vi "Abgleich_Finetuning.vi"(0 "DAQ Settings":T1={"sampling rate [Hz]"=50000.0, "actual update rate"=50000.00001018634, "output physical channel"="SOUNDACQ/ao0", "input channel (stimulus)"="SOUNDACQ/ai0", "propagation delay [samples]"=133, "input channel (response)"="SOUNDACQ/ai1"} {"propagation delay [samples]" min=1 step=1; "actual update rate" format="%.2f"; "sampling rate [Hz]" format="%.2f"}, 1 "Soll_Pegel(dBSPL)":i32=-1, 5 "FRF Settings":T3={"window"=1, "block size"=1000, "view"={"dB On"=TRUE, "unwrap phase"=FALSE, "convert to degree"=TRUE}, "averaging parameters"={"averaging mode"=enum."RMS averaging", "weighting mode"=enum."Exponential", "number of averages"=2, "linear mode"=enum."One shot"}, "restart averaging"=FALSE} {"averaging parameters"."number of averages" min=1 step=1; "block size" min=128; "window" items=["None"=0, "Hanning"=1, "Hamming"=2, "Blackman-Harris"=3, "Exact Blackman"=4, "Blackman"=5, "Flat Top"=6, "4 Term B-Harris "=7, "7 Term B-Harris"=8, "Low Sidelobe"=9, "Force - Exponential"=10, "Blackman Nuttall"=11, "Triangle"=30, "Bartlett-Hanning"=31, "Bohman"=32, "Parzen"=33, "Welch"=34, "Kaiser"=60, "Dolph-Chebyshev"=61, "Gaussian"=62]}, 7 "frequency":dbl=1000.0, 9 "sensitivity(mV/Pa)":dbl=336.0, 11 "error in":errorcluster, 12 "Start_Amplitude(V)":dbl=0.605 min=0.0 format="%.3f") -> (4 "End_Amplitude(V)":dbl=0.605 min=0.0 format="%.3f", 6 "Ist_Pegel(dBSPL)":dbl=94.02694316227692, 8 "detected fund. amp.":dbl=0.47778380964100664 format="%.5f", 15 "error out":errorcluster)   [LabVIEW 2018]
uses:
  <vilib>/addons/_NISVFA/_Shared subVIs/Controls/svc_Window [Dual FFT].ctl
  <vilib>/DAQmx/write.llb/DAQmx Write (Analog 1D DBL 1Chan NSamp).vi
  <vilib>/DAQmx/read.llb/DAQmx Read (Analog 1D Wfm NChan NSamp).vi
  <vilib>/DAQmx/create/channels.llb/DAQmx Create Channel (AI-Voltage-Basic).vi
  <vilib>/DAQmx/configure/timing.llb/DAQmx Timing (Sample Clock).vi
  <vilib>/DAQmx/create/channels.llb/DAQmx Create Channel (AO-Voltage-Basic).vi
  <vilib>/DAQmx/configure/trigger.llb/DAQmx Start Trigger (Digital Edge).vi
  <vilib>/DAQmx/miscellaneous.llb/DAQmx Fill In Error Info.vi
  <vilib>/addons/_NISVFA/_Baseband FFT/SVFA Frequency Response (1x1) (Mag-Phase).vi
  <vilib>/addons/Sound and Vibration/svt_Distortion/SVT THD and Harmonic Components (Time) (1 Ch).vi
  <vilib>/addons/_NISVFA/_Baseband FFT/SVFA Power Spectrum (1 Ch).vi
  <vilib>/Analysis/NI_AALBase.lvlib
  <vilib>/addons/Sound and Vibration/svt_Distortion/SoundVib_Distortion.lvlib
  <resource>/objmgr/daqmx.rc
panel:
  out "fr1000Hz":dbl(graph)=999.9999374706828
  out "mean":dbl=0.501952560805785
  out "standard deviation":dbl=0.010795190304670955
  out "Array":u32[](array[numeric])
  out "Ist_Pegel(dBSPL) Time Chart":cluster{dbl[], dbl[]}[](graph)
  in  "Coh Faktor Thresold":dbl=999.98 format="%#_10g"
  out "Filtered FR_Time Chart":cluster{dbl[], dbl[]}(graph)
  out "Big Sound Disturbances detected":i32=1
  out "Sound Pressure (Pa)":dbl=1.0054886063639832
  in  "swept sine settings":enum32{"DAQ Settings", "FRF Settings"}(tab)
  in  "input channel (response)":tag="SOUNDACQ/ai1"
  in  "propagation delay [samples]":i32=133 min=1 step=1
  in  "input channel (stimulus)":tag="SOUNDACQ/ai0"
  in  "output physical channel":tag="SOUNDACQ/ao0"
  out "actual update rate":dbl=50000.00001018634 format="%.2f"
  in  "sampling rate [Hz]":dbl=50000.0 format="%.2f"
  out "averages completed":dbl=4358.0
  in  "restart averaging":bool
  in  "averaging parameters":T4={"averaging mode"=enum."RMS averaging", "weighting mode"=enum."Exponential", "number of averages"=2, "linear mode"=enum."One shot"} {"number of averages" min=1 step=1}
  in  "view":T5={"dB On"=TRUE, "unwrap phase"=FALSE, "convert to degree"=TRUE}
  in  "block size":i32=1000 min=128
  in  "window":T2=1 items=["None"=0, "Hanning"=1, "Hamming"=2, "Blackman-Harris"=3, "Exact Blackman"=4, "Blackman"=5, "Flat Top"=6, "4 Term B-Harris "=7, "7 Term B-Harris"=8, "Low Sidelobe"=9, "Force - Exponential"=10, "Blackman Nuttall"=11, "Triangle"=30, "Bartlett-Hanning"=31, "Bohman"=32, "Parzen"=33, "Welch"=34, "Kaiser"=60, "Dolph-Chebyshev"=61, "Gaussian"=62]
  in  "Tab Control":enum32{"Getting Started", "Time Record", "FRF"}(tab)=enum."FRF"
  in  "Getting Started Text":string="GETTING STARTED\n\nThis VI measures the Frequency Response Function (FRF) of a device under test (DUT).  It generates a broadband stimulus signal to excite the DUT.  The magnitude and phase of the DUT output are compared to the stimulus signal to calculate the FRF.  \n\nRefer to the wiring diagram to physically connect the DSA or DAQ device to the DUT.  This example uses two analog input channels and one analog output channel.  Note that the analog output is connected to both the DUT input and to the first analog input channel on the measurement device.  \n\nThe wiring diagram assumes that you use the default channel settings.  If you change the channel settings in the VI front panel you should adjust the physical connections appropriately.\n\nNI strongly recommends that you take precautions to limit the effects of out-of-band aliasing in your frequency domain measurements.  DSA devices use transparent digital and analog hardware filtering to eliminate aliased input and output frequencies.  Multifunction DAQ devices are more susceptible to the effects of aliased frequencies.  If you are using a non-DSA measurement device, we recommend addressing potential aliasing through high sampling rates, built-in analog filters on S Series devices, and/or external analog filters.\n\n\nKEY PARAMETERS\n\nDAQ Configuration:  device propagation delay [samples]\n\nThis parameter quantifies the time, measured in sample intervals, between when a sample of data is generated on analog output and when it is read on the analog input.  Common sources of delay are analog or digital filters and propagation time for acoustical or mechanical signals.  The combined delay of the digital anti-aliasing and anti-imaging filters on the NI PCI-4451 and PCI-4551 devices is approximately 77 samples.  When using a multifunction E Series or S Series device, we recommend entering a delay of 1 sample.  An easy way to determine this delay for any given measurement system is to run SVT Measure Propagation Delay.vi.  This VI is available from the LabVIEW Functions palette under Sound and Vibration >> Calibration.\n\n\nSource Settings:  signal type\n\nThis control allows you to specify the type of stimulus signal you would like to generate.  All of the available signal sources are broadband stimuli with frequency content ranging from just above DC to the value specified in the \"Maximum Frequency of Interest\" control.  Note that if you use the \"Chirp\" or \"Frequency flat chirp\" signal types, you should select \"None\" for the window type.\n\nSource Settings:  maximum frequency of interest [Hz]\n\nThis setting controls the sampling rate for input and output.  The sampling rate is 2.5 times the value of this control.  Reducing the maximum frequency of interest may help if you encounter issues of data transfer bandwidth.\n\nMeasurement Settings:  frequency resolution [Hz]\n\nThis setting controls the width of a single frequency bin in the frequency response measurement.  Improving the frequency resolution requires more data points per average. Thus, the acquisition block size increases with finer frequency resolutions.  Improving (i.e. reducing) the frequency resolution may help if you encounter issues of data transfer bandwidth. \n\nMeasurement Settings:  window\n\nThis setting controls the time-domain window applied to the input signals before the frequency response function is calculated.  If you use the \"Chirp\" or \"Frequency flat chirp\" excitation types, you should not apply a window.\n\n\nMeasurement Settings:  settle time [s]\n\nThis control allows you to specify a time interval between when the stimulus generation starts and when the measurement actually begins. This time interval will be coerced to an integer number of data blocks.  If your DUT has a significant transient response to the start of a stimulus signal, select the appropriate settle time to allow this transient response to pass.\n"
  out "time record 2":waveform(dbl)[](graph)=[{"t0"=timestamp(3564665204.4424295 s since 1904-01-01), "dt"=1.9999999995925458e-05, "Y"=array[1000 elements], "attributes"=variant("NI_ChannelName"=variant(string "stimulus"), "NI_UnitDescription"=variant(string "Volts"))}, {"t0"=timestamp(3564665204.4424295 s since 1904-01-01), "dt"=1.9999999995925458e-05, "Y"=array[1000 elements], "attributes"=variant("NI_ChannelName"=variant(string "response"), "NI_UnitDescription"=variant(string "Volts"))}]
  out "Waveform Graph":dbl[](graph)=[0.0, 0.07582660630640407, 0.15045738173473716, 0.22271535437423018, 0.29146097283153777, 0.35561007763694624, 0.4141509990868567, 0.4661605118793525, 0.5108183949287192, 0.5474203667419418, 0.5753891923585679, 0.5942837866908567, 0.6038061706991042, 0.6038061706991044, 0.5942837866908566, 0.5753891923585679, 0.5474203667419417, 0.510818394928719, 0.46616051187935237, 0.41415099908685654, 0.35561007763694613, 0.2914609728315376, 0.22271535437423004, 0.15045738173473697, 0.07582660630640392, -2.0721814021629203e-16, -0.07582660630640423, -0.15045738173473736, -0.22271535437423032, -0.29146097283153793, -0.35561007763694635, -0.4141509990868568, -0.4661605118793526, -0.5108183949287193, -0.5474203667419418, -0.575389192358568, -0.5942837866908566, -0.6038061706991044, -0.6038061706991041, -0.5942837866908567, -0.5753891923585677, -0.5474203667419417, -0.5108183949287188, -0.4661605118793523, -0.4141509990868563, -0.35561007763694596, -0.2914609728315374, -0.22271535437422982, -0.1504573817347368, -0.07582660630640367, 3.226585665316861e-16, 0.07582660630640449, 0.15045738173473744, 0.2227153543742306, 0.291460972831538, 0.35561007763694663, 0.4141509990868568, 0.4661605118793528, 0.5108183949287192, 0.547420366741942, 0.5753891923585679, 0.5942837866908568, 0.6038061706991041, 0.6038061706991044, 0.5942837866908564, 0.5753891923585679, 0.5474203667419414, 0.5108183949287189, 0.466160511879352, 0.4141509990868563, 0.3556100776369457, 0.29146097283153727, 0.2227153543742296, 0.15045738173473658, 0.0758266063064035, -6.342176133225519e-16, -0.07582660630640459, -0.1504573817347378, -0.22271535437423062, -0.2914609728315384, -0.3556100776369466, -0.4141509990868572, -0.4661605118793527, -0.5108183949287196, -0.5474203667419418, -0.5753891923585682, -0.5942837866908565, -0.6038061706991045, -0.6038061706991039, -0.5942837866908567, -0.5753891923585674, -0.5474203667419416, -0.5108183949287185, -0.4661605118793521, -0.41415099908685593, -0.3556100776369457, -0.291460972831537, -0.22271535437422946, -0.15045738173473638, -0.07582660630640327, 7.187176201406409e-16, 0.07582660630640492, 0.15045738173473777, 0.222715354374231, 0.2914609728315382, 0.355610077636947, 0.41415099908685693, 0.46616051187935315, 0.5108183949287192, 0.5474203667419423, 0.5753891923585678, 0.5942837866908569, 0.6038061706991039, 0.6038061706991044, 0.5942837866908561, 0.5753891923585678, 0.5474203667419412, 0.5108183949287187, 0.4661605118793517, 0.41415099908685604, 0.3556100776369454, 0.29146097283153694, 0.2227153543742293, 0.15045738173473622, 0.07582660630640321, -1.0083893355744555e-15, -0.07582660630640485, -0.15045738173473816, -0.22271535437423082, -0.2914609728315387, -0.35561007763694674, -0.4141509990868575, -0.46616051187935276, -0.5108183949287198, -0.5474203667419418, -0.5753891923585684, -0.5942837866908565, -0.6038061706991046, -0.6038061706991039, -0.5942837866908567, -0.5753891923585673, -0.5474203667419415, -0.5108183949287184, -0.46616051187935187, -0.41415099908685576, -0.35561007763694535, -0.29146097283153677, -0.22271535437422907, -0.15045738173473613, -0.07582660630640284, 9.913809139935892e-16, 0.07582660630640536, 0.15045738173473805, 0.22271535437423143, 0.2914609728315385, 0.3556100776369474, 0.4141509990868572, 0.4661605118793535, 0.5108183949287195, 0.5474203667419426, 0.575389192358568, 0.5942837866908571, 0.6038061706991041, 0.6038061706991045, 0.5942837866908562, 0.5753891923585678, 0.5474203667419412, 0.5108183949287186, 0.4661605118793516, 0.4141509990868558, 0.3556100776369452, 0.2914609728315366, 0.22271535437422899, 0.15045738173473577, 0.07582660630640285, -1.5111745405374521e-15, -0.07582660630640525, -0.1504573817347387, -0.22271535437423123, -0.2914609728315392, -0.35561007763694713, -0.414150999086858, -0.46616051187935315, -0.5108183949287202, -0.5474203667419422, -0.5753891923585687, -0.5942837866908567, -0.6038061706991047, -0.603806170699104, -0.5942837866908567, -0.5753891923585673, -0.5474203667419414, -0.5108183949287183, -0.46616051187935165, -0.41415099908685554, -0.3556100776369451, -0.29146097283153644, -0.22271535437422874, -0.15045738173473575, -0.07582660630640245, 1.416211982754878e-15, 0.07582660630640578, 0.1504573817347385, 0.22271535437423184, 0.29146097283153893, 0.3556100776369478, 0.4141509990868576, 0.4661605118793538, 0.5108183949287197, 0.5474203667419428, 0.5753891923585681, 0.5942837866908572, 0.6038061706991041, 0.6038061706991045, 0.5942837866908561, 0.5753891923585677, 0.547420366741941, 0.5108183949287184, 0.4661605118793513, 0.4141509990868555, 0.35561007763694485, 0.2914609728315362, 0.22271535437422862, 0.15045738173473538, 0.07582660630640248, -1.900714828584338e-15, -0.07582660630640561, -0.15045738173473908, -0.22271535437423157, -0.29146097283153954, -0.3556100776369474, -0.4141509990868582, -0.4661605118793533, -0.5108183949287204, -0.5474203667419423, -0.5753891923585688, -0.5942837866908567, -0.6038061706991047, -0.6038061706991039, -0.5942837866908566, -0.5753891923585671, -0.5474203667419413, -0.510818394928718, -0.4661605118793515, -0.41415099908685515, -0.3556100776369448, -0.29146097283153605, -0.22271535437422837, -0.15045738173473536, -0.07582660630640205, 1.7820489008057994e-15, 0.0758266063064062, 0.1504573817347388, 0.22271535437423226, 0.29146097283153916, 0.3556100776369482, 0.41415099908685776, 0.46616051187935414, 0.5108183949287198, 0.547420366741943, 0.5753891923585682, 0.5942837866908574, 0.6038061706991041, 0.6038061706991045, 0.594283786690856, 0.5753891923585676, 0.5474203667419407, 0.5108183949287183, 0.46616051187935104, 0.4141509990868553, 0.3556100776369445, 0.291460972831536, 0.22271535437422826, 0.15045738173473508, 0.07582660630640209, -2.2531754023322192e-15, -0.075826606306406, -0.15045738173473944, -0.22271535437423193, -0.29146097283153993, -0.35561007763694774, -0.4141509990868586, -0.4661605118793536, -0.5108183949287207, -0.5474203667419425, -0.575389192358569, -0.5942837866908568, -0.6038061706991048, -0.6038061706991039, -0.5942837866908566, -0.575389192358567, -0.5474203667419412, -0.5108183949287177, -0.46616051187935126, -0.4141509990868549, -0.3556100776369445, -0.2914609728315357, -0.22271535437422804, -0.15045738173473497, -0.07582660630640169, 2.196430971129759e-15, 0.07582660630640656, 0.15045738173473922, 0.2227153543742326, 0.29146097283153954, 0.35561007763694846, 0.4141509990868581, 0.46616051187935437, 0.51081839492872, 0.5474203667419433, 0.5753891923585683, 0.5942837866908576, 0.6038061706991041, 0.6038061706991046, 0.5942837866908559, 0.5753891923585676, 0.5474203667419405, 0.5108183949287182, 0.4661605118793507, 0.4141509990868551, 0.35561007763694413, 0.2914609728315357, 0.22271535437422785, 0.15045738173473475, 0.07582660630640167, -2.6303828906670823e-15, -0.07582660630640639, -0.15045738173473985, -0.22271535437423226, -0.2914609728315403, -0.35561007763694796, -0.41415099908685893, -0.46616051187935376, -0.5108183949287209, -0.5474203667419425, -0.5753891923585692, -0.5942837866908567, -0.603806170699105, -0.6038061706991037, -0.5942837866908567, -0.5753891923585667, -0.5474203667419412, -0.5108183949287174, -0.46616051187935115, -0.4141509990868545, -0.3556100776369443, -0.29146097283153527, -0.22271535437422776, -0.15045738173473455, -0.07582660630640135, 2.5672010090654895e-15, 0.07582660630640693, 0.15045738173473952, 0.222715354374233, 0.29146097283153977, 0.35561007763694885, 0.4141509990868582, 0.4661605118793547, 0.51081839492872, 0.5474203667419435, 0.5753891923585682, 0.5942837866908577, 0.6038061706991039, 0.6038061706991046, 0.5942837866908556, 0.5753891923585674, 0.5474203667419402, 0.510818394928718, 0.46616051187935037, 0.4141509990868548, 0.35561007763694374, 0.2914609728315354, 0.22271535437422746, 0.15045738173473439, 0.07582660630640131, -2.984632397999565e-15, -0.0758266063064067, -0.15045738173474016, -0.2227153543742325, -0.2914609728315406, -0.35561007763694813, -0.41415099908685915, -0.4661605118793538, -0.5108183949287212, -0.5474203667419425, -0.5753891923585693, -0.5942837866908567, -0.603806170699105, -0.6038061706991036, -0.5942837866908566, -0.5753891923585666, -0.547420366741941, -0.5108183949287172, -0.46616051187935087, -0.4141509990868542, -0.35561007763694397, -0.291460972831535, -0.22271535437422738, -0.15045738173473422, -0.07582660630640094, 2.911624934209822e-15, 0.07582660630640733, 0.15045738173473985, 0.22271535437423337, 0.2914609728315401, 0.3556100776369492, 0.4141509990868585, 0.466160511879355, 0.5108183949287203, 0.5474203667419437, 0.5753891923585683, 0.5942837866908578, 0.6038061706991039, 0.6038061706991046, 0.5942837866908556, 0.5753891923585673, 0.5474203667419401, 0.5108183949287177, 0.46616051187935015, 0.4141509990868545, 0.35561007763694347, 0.291460972831535, 0.22271535437422713, 0.15045738173473394, 0.07582660630640095, -3.45132722314595e-15, -0.07582660630640707, -0.15045738173474063, -0.22271535437423287, -0.29146097283154104, -0.35561007763694846, -0.41415099908685954, -0.4661605118793541, -0.5108183949287214, -0.5474203667419427, -0.5753891923585694, -0.5942837866908568, -0.603806170699105, -0.6038061706991036, -0.5942837866908565, -0.5753891923585664, -0.5474203667419407, -0.510818394928717, -0.46616051187935054, -0.41415099908685393, -0.3556100776369436, -0.29146097283153466, -0.22271535437422696, -0.15045738173473386, -0.0758266063064005, 3.28743651224761e-15, 0.07582660630640777, 0.15045738173474021, 0.22271535437423376, 0.29146097283154043, 0.3556100776369495, 0.41415099908685876, 0.4661605118793552, 0.5108183949287205, 0.5474203667419438, 0.5753891923585684, 0.5942837866908578, 0.603806170699104, 0.6038061706991045, 0.5942837866908556, 0.5753891923585671, 0.54742036674194, 0.5108183949287174, 0.4661605118793499, 0.4141509990868541, 0.3556100776369432, 0.29146097283153455, 0.2227153543742268, 0.1504573817347335, 0.07582660630640058, -3.876510657613297e-15, -0.07582660630640746, -0.15045738173474102, -0.22271535437423323, -0.2914609728315414, -0.3556100776369488, -0.41415099908685976, -0.46616051187935437, -0.5108183949287215, -0.5474203667419429, -0.5753891923585694, -0.5942837866908569, -0.6038061706991049, -0.6038061706991037, -0.5942837866908562, -0.5753891923585664, -0.5474203667419404, -0.5108183949287168, -0.46616051187935015, -0.4141509990868537, -0.35561007763694313, -0.2914609728315343, -0.2227153543742265, -0.15045738173473347, -0.07582660630640005, 3.708391558242263e-15, 0.07582660630640818, 0.15045738173474066, 0.22271535437423412, 0.2914609728315408, 0.3556100776369498, 0.4141509990868591, 0.46616051187935537, 0.5108183949287208, 0.5474203667419438, 0.5753891923585688, 0.5942837866908577, 0.6038061706991042, 0.6038061706991042, 0.5942837866908557, 0.5753891923585668, 0.54742036674194, 0.5108183949287171, 0.4661605118793498, 0.4141509990868537, 0.3556100776369429, 0.2914609728315341, 0.2227153543742264, 0.15045738173473305, 0.0758266063064001, -4.295026248719858e-15, -0.07582660630640799, -0.15045738173474138, -0.2227153543742338, -0.29146097283154165, -0.35561007763694935, -0.41415099908686, -0.46616051187935487, -0.5108183949287216, -0.5474203667419433, -0.5753891923585694, -0.5942837866908571, -0.6038061706991048, -0.6038061706991038, -0.594283786690856, -0.5753891923585664, -0.5474203667419401, -0.5108183949287167, -0.46616051187934976, -0.4141509990868535, -0.3556100776369427, -0.291460972831534, -0.22271535437422602, -0.15045738173473305, -0.07582660630639959, 4.18118502060888e-15, 0.0758266063064086, 0.15045738173474116, 0.22271535437423445, 0.2914609728315413, 0.35561007763695, 0.4141509990868596, 0.46616051187935553, 0.5108183949287213, 0.5474203667419439, 0.5753891923585691, 0.5942837866908577, 0.6038061706991045, 0.6038061706991041, 0.5942837866908557, 0.5753891923585666, 0.5474203667419398, 0.5108183949287167, 0.4661605118793496, 0.4141509990868533, 0.3556100776369426, 0.29146097283153366, 0.222715354374226, 0.15045738173473258, 0.07582660630639963, -4.7612196303614684e-15, -0.07582660630640849, -0.1504573817347418, -0.2227153543742343, -0.291460972831542, -0.3556100776369498, -0.4141509990868602, -0.46616051187935525, -0.5108183949287218, -0.5474203667419436, -0.5753891923585696, -0.5942837866908574, -0.6038061706991048, -0.6038061706991038, -0.5942837866908559, -0.5753891923585663, -0.5474203667419398, -0.5108183949287165, -0.4661605118793494, -0.41415099908685316, -0.3556100776369423, -0.2914609728315336, -0.22271535437422557, -0.1504573817347326, -0.07582660630639912, 4.6485710246402245e-15, 0.07582660630640906, 0.1504573817347416, 0.22271535437423487, 0.2914609728315417, 0.35561007763695035, 0.4141509990868599, 0.46616051187935575, 0.5108183949287214, 0.547420366741944, 0.5753891923585691, 0.5942837866908577, 0.6038061706991044, 0.603806170699104, 0.5942837866908556, 0.5753891923585663, 0.5474203667419396, 0.5108183949287164, 0.4661605118793493, 0.41415099908685293, 0.3556100776369423, 0.29146097283153327, 0.22271535437422568, 0.1504573817347322, 0.07582660630639933, -5.138386461114863e-15, -0.07582660630640878, -0.15045738173474216, -0.22271535437423454, -0.2914609728315423, -0.35561007763695, -0.4141509990868605, -0.4661605118793554, -0.5108183949287219, -0.5474203667419437, -0.5753891923585696, -0.5942837866908574, -0.6038061706991047, -0.6038061706991038, -0.5942837866908557, -0.5753891923585662, -0.5474203667419396, -0.5108183949287164, -0.46616051187934915, -0.414150999086853, -0.35561007763694197, -0.2914609728315334, -0.2227153543742252, -0.15045738173473236, -0.07582660630639876, 4.928037687125519e-15, 0.0758266063064094, 0.1504573817347419, 0.2227153543742352, 0.29146097283154204, 0.35561007763695063, 0.4141509990868602, 0.466160511879356, 0.5108183949287217, 0.5474203667419442, 0.5753891923585693, 0.5942837866908577, 0.6038061706991045, 0.6038061706991039, 0.5942837866908556, 0.5753891923585662, 0.5474203667419395, 0.5108183949287162, 0.4661605118793491, 0.4141509990868526, 0.355610077636942, 0.2914609728315329, 0.22271535437422535, 0.15045738173473178, 0.07582660630639895, -5.5518740646465226e-15, -0.07582660630640915, -0.15045738173474252, -0.2227153543742349, -0.2914609728315426, -0.35561007763695035, -0.4141509990868607, -0.4661605118793557, -0.510818394928722, -0.5474203667419439, -0.5753891923585696, -0.5942837866908576, -0.6038061706991046, -0.6038061706991039, -0.5942837866908556, -0.5753891923585662, -0.5474203667419394, -0.5108183949287163, -0.46616051187934887, -0.41415099908685277, -0.35561007763694163, -0.29146097283153305, -0.22271535437422488, -0.15045738173473194, -0.07582660630639841, 5.387861381003778e-15, 0.07582660630640974, 0.15045738173474238, 0.22271535437423548, 0.2914609728315425, 0.35561007763695085, 0.4141509990868606, 0.4661605118793561, 0.510818394928722, 0.5474203667419442, 0.5753891923585696, 0.5942837866908577, 0.6038061706991046, 0.6038061706991039, 0.5942837866908556, 0.5753891923585661, 0.5474203667419394, 0.5108183949287161, 0.46616051187934887, 0.41415099908685243, 0.3556100776369417, 0.29146097283153266, 0.22271535437422496, 0.1504573817347315, 0.07582660630639852, -5.8520354360991345e-15, -0.0758266063064096, -0.15045738173474282, -0.22271535437423534, -0.2914609728315429, -0.35561007763695074, -0.4141509990868609, -0.46616051187935603, -0.5108183949287223, -0.5474203667419442, -0.5753891923585698, -0.5942837866908577, -0.6038061706991047, -0.6038061706991039, -0.5942837866908556, -0.5753891923585661, -0.5474203667419393, -0.5108183949287161, -0.46616051187934865, -0.41415099908685243, -0.35561007763694136, -0.29146097283153266, -0.22271535437422454, -0.15045738173473153, -0.07582660630639806, 5.817937277774465e-15, 0.07582660630641008, 0.1504573817347428, 0.2227153543742358, 0.2914609728315429, 0.3556100776369512, 0.4141509990868609, 0.46616051187935637, 0.5108183949287223, 0.5474203667419444, 0.5753891923585698, 0.5942837866908578, 0.6038061706991047, 0.6038061706991039, 0.5942837866908556, 0.575389192358566, 0.5474203667419393, 0.5108183949287158, 0.46616051187934865, 0.41415099908685216, 0.35561007763694136, 0.29146097283153233, 0.22271535437422454, 0.15045738173473114, 0.07582660630639806, -6.232305795571269e-15, -0.07582660630641008, -0.1504573817347432, -0.2227153543742358, -0.29146097283154326, -0.3556100776369512, -0.41415099908686126, -0.46616051187935637, -0.5108183949287225, -0.5474203667419444, -0.5753891923585699, -0.5942837866908578, -0.6038061706991047, -0.6038061706991039, -0.5942837866908555, -0.575389192358566, -0.5474203667419392, -0.5108183949287158, -0.4661605118793485, -0.41415099908685216, -0.35561007763694114, -0.29146097283153233, -0.22271535437422427, -0.15045738173473114, -0.07582660630639775, 6.229866340683177e-15, 0.07582660630641042, 0.1504573817347432, 0.22271535437423615, 0.29146097283154326, 0.35561007763695146, 0.41415099908686126, 0.46616051187935664, 0.5108183949287225, 0.5474203667419446, 0.5753891923585699, 0.5942837866908579, 0.6038061706991047, 0.6038061706991039, 0.5942837866908555, 0.5753891923585659, 0.5474203667419391, 0.5108183949287156, 0.46616051187934837, 0.4141509990868519, 0.355610077636941, 0.291460972831532, 0.22271535437422418, 0.15045738173473078, 0.07582660630639769, -6.589550411405243e-15, -0.07582660630641044, -0.15045738173474354, -0.22271535437423615, -0.29146097283154354, -0.35561007763695146, -0.4141509990868615, -0.4661605118793566, -0.5108183949287227, -0.5474203667419445, -0.57538919235857, -0.5942837866908578, -0.6038061706991047, -0.6038061706991038, -0.5942837866908554, -0.5753891923585658, -0.547420366741939, -0.5108183949287155, -0.4661605118793482, -0.41415099908685177, -0.3556100776369408, -0.2914609728315319, -0.22271535437422388, -0.1504573817347307, -0.07582660630639734, 6.644383936278697e-15, 0.07582660630641082, 0.15045738173474357, 0.2227153543742365, 0.29146097283154354, 0.3556100776369518, 0.4141509990868614, 0.46616051187935686, 0.5108183949287226, 0.5474203667419447, 0.5753891923585699, 0.5942837866908579, 0.6038061706991046, 0.6038061706991038, 0.5942837866908552, 0.5753891923585657, 0.5474203667419388, 0.5108183949287153, 0.4661605118793481, 0.4141509990868515, 0.3556100776369407, 0.29146097283153155, 0.2227153543742238, 0.15045738173473033, 0.07582660630639729, -7.011115321121919e-15, -0.07582660630641085, -0.1504573817347439, -0.2227153543742365, -0.2914609728315438, -0.35561007763695174, -0.41415099908686165, -0.4661605118793568, -0.5108183949287227, -0.5474203667419447, -0.5753891923585699, -0.5942837866908579, -0.6038061706991046, -0.6038061706991038, -0.5942837866908551, -0.5753891923585657, -0.5474203667419386, -0.5108183949287153, -0.4661605118793478, -0.41415099908685143, -0.35561007763694036, -0.2914609728315315, -0.22271535437422346, -0.15045738173473025, -0.07582660630639695, 7.1043702604828285e-15, 0.07582660630641115, 0.15045738173474402, 0.22271535437423676, 0.29146097283154393, 0.35561007763695196, 0.41415099908686176, 0.4661605118793569, 0.5108183949287228, 0.5474203667419447, 0.57538919235857, 0.5942837866908578, 0.6038061706991046, 0.6038061706991036, 0.5942837866908551, 0.5753891923585654, 0.5474203667419386, 0.5108183949287151, 0.46616051187934776, 0.4141509990868512, 0.3556100776369403, 0.2914609728315313, 0.22271535437422338, 0.15045738173473003, 0.07582660630639686, -7.316250470040808e-15, -0.07582660630641126, -0.1504573817347442, -0.2227153543742369, -0.2914609728315441, -0.35561007763695207, -0.41415099908686187, -0.46616051187935703, -0.5108183949287229, -0.5474203667419448, -0.57538919235857, -0.5942837866908579, -0.6038061706991046, -0.6038061706991037, -0.5942837866908551, -0.5753891923585654, -0.5474203667419385, -0.510818394928715, -0.4661605118793476, -0.41415099908685105, -0.3556100776369401, -0.29146097283153105, -0.22271535437422313, -0.1504573817347298, -0.0758266063063966, 7.531125788100279e-15, 0.07582660630641153, 0.1504573817347444, 0.22271535437423712, 0.29146097283154426, 0.35561007763695224, 0.41415099908686204, 0.46616051187935714, 0.510818394928723, 0.5474203667419448, 0.5753891923585701, 0.5942837866908579, 0.6038061706991046, 0.6038061706991037, 0.594283786690855, 0.5753891923585654, 0.5474203667419384, 0.510818394928715, 0.46616051187934743, 0.414150999086851, 0.35561007763693986, 0.291460972831531, 0.22271535437422288, 0.1504573817347297, 0.07582660630639633, -7.679661485730793e-15, -0.07582660630641178, -0.15045738173474457, -0.22271535437423737, -0.29146097283154443, -0.35561007763695246, -0.4141509990868622, -0.46616051187935736, -0.5108183949287232, -0.547420366741945, -0.5753891923585702, -0.594283786690858, -0.6038061706991047, -0.6038061706991037, -0.5942837866908551, -0.5753891923585653, -0.5474203667419384, -0.5108183949287147, -0.46616051187934743, -0.4141509990868507, -0.35561007763693986, -0.29146097283153066, -0.22271535437422282, -0.15045738173472936, -0.07582660630639625]
  out "phase":cluster{"f0":dbl, "df":dbl, "magnitude":dbl[]}(graph)={"f0"=0.0, "df"=50.000000010186355, "magnitude"=[180.0, -172.64056285116183, 36.88310703154806, 172.78407319533684, -42.69926621349432, -37.71150503639981, -121.44831900984987, -149.89743852578755, -170.87471452410773, 155.8203013631222, 165.984586805478, -93.20548927993258, -16.38559101191221, 21.71918430421371, 104.7991460775427, 91.9430956170447, 31.838335606486094, -114.31546941063381, 142.08668104635598, 6.739071255993011, 6.759732009788827, 6.7871846639981985, 94.74880045442791, 14.3265311512339, 27.889138437499792, 73.24572171654467, 65.50798237157126, 43.127329104588554, 59.73975162771791, 72.13808243854464, 36.56171129466196, -20.108878066709405, -54.59109000609955, -129.06888609478054, 69.0795671549659, 126.01943511916947, -88.59765097828873, 110.14295663657549, -144.55045917574864, -72.67096102208038, -49.90185295440582, -37.076592009573694, -16.40566149978067, -85.22268677969943, -4.9295395687997745, 22.967986998276366, -41.97149388778875, -80.67166596658599, 114.23744657415926, 165.106276799966, -120.18224973807366, 11.717525036896758, 2.676916857080053, 32.79063411325977, 39.02484429698921, 3.8396679362312396, -36.24092021684923, -37.53321412302254, 30.56108836514342, -119.3583245223785, -112.05698012215514, -92.18372126012834, -34.51007793765087, -3.1280626709700154, 80.05656827421672, 116.17934917101998, 117.02668298124925, 34.116401495673735, 136.1715580455397, -121.98752711321339, -86.82126019616544, -178.64989935559964, 115.59590672624017, -85.1129540254658, 134.45752403802035, -5.888018676520777, -118.3702050407098, 149.83595773265435, 18.99897497952458, 3.4516847947770137, -45.96737658560425, -5.213584668563267, 153.63146902508265, 139.29971463458878, -66.36298594036064, -175.8034531681047, 164.3846644216621, 86.35934015566158, 112.09593761171207, -90.39808756531778, -162.91803204617213, 167.30525341540556, 124.7614876739556, 121.78806219109215, 54.947649494611845, -71.92305306617722, -15.964839625601556, 114.49256191875354, 156.95055916020087, -88.48116391944549, -170.51610028754166, -39.64936418511651, -135.541354224487, -176.43262194381964, 68.00461771196568, 132.79650459823657, 125.19347433611661, 106.86209026259567, 47.660456974457105, 135.00417570286928, 178.4553866934091, 155.55638021037504, 95.7978967647022, 171.54241526421447, 179.7985898148362, -95.15134197474572, 160.0235287302262, 159.60365368473774, 176.9185863486146, -175.4881884518036, -175.4306810275502, -167.33427938697974, -25.61120668934921, -51.70852592291764, 126.9304971283637, 101.8029328686014, 113.83159264234129, 84.44642798350459, 54.18984060175027, 136.65253617284367, 44.11793870955932, 40.69200562246512, 122.62904192236984, 90.76813617839233, 17.146191015200696, -154.119257547954, 143.98232588509015, 151.68812121298896, 143.7088478722457, 151.48105319683006, 120.18716562214689, -20.156156044570604, -28.842650378456717, 12.700226669500298, 57.24577206952305, 134.62525045957042, 132.31803568796687, 100.60735967567746, 87.59460845017458, 166.8776219006705, 29.408145748594695, -44.54317351601723, -116.600456480295, 131.47984689081812, 69.22513284563804, 34.553555199160115, 8.103459457681609, -133.28650832776043, 21.428660815764708, 59.98506178056983, 75.58999805175641, 154.44034054458302, 164.52328405418635, 95.06910518946928, 84.68298639861172, -2.7953014030864654, -32.04528210692494, -114.93599718798703, -175.22895976598014, 177.03593219823682, -76.06171969866125, 72.60596987752568, 106.37879356773945, -46.42455902861751, 5.433365073946909, 1.2260214470119852, 30.773824434255555, 96.15773439526127, 164.9918567050007, -135.70942827811513, -136.32850812434148, 50.2271069491322, 28.192918376421233, 63.4572126217022, 67.53491106183209, 74.54694777973546, 76.09363804294094, 51.28457026815978, 69.1905665229993, -124.00788104795676, 162.87689127542777, 111.83791599021562, -4.763285824074514, -43.327868111460475, -57.83504816321683, -42.70803520414571, -41.109785068639866, -42.42709426873382, -7.396287452847097, -64.60304462884548, -164.4326354370841, 24.589814075745572, 0.26296607302483244, 123.61511234720113, 99.49835611869776, 96.7722790778152, 147.92060549519377, -25.019265737063506, 32.89659715264034, -59.12588433702089, -67.51690420180572, 47.40049831543473, 115.14534533644922, -157.16673180753492, 159.2090367687523, 24.569206584467945, -169.14148485623244, 50.861348129921566, 137.69889668166354, -154.00913262810747, 96.44361857559161, 49.72039989882201, -118.03881167127318, 170.21614075625618, -5.937849562108772, -14.09488578493923, -27.86637409890263, -41.02514087379638, -91.82996101850388, -8.242496862104364, -61.3635103463718, -166.7381438632079, 144.55058317242776, -52.6703810780514, 8.960830934654682, -109.86956104060425, 79.70386810020958, -6.53750799691418, 64.03594493965618, 115.1088831309143, 159.50925260857406, 114.83781958681269, 92.5108612902118, -114.10021750708138, 126.51559895610096, 101.56351773475396, 10.433846609317126, 33.22018997987736, 96.98387889904645, -71.46958580328469, 88.79983010314018, 157.06885666356436, 159.15319251265393, 113.86815321159554, 28.63894492949662, 25.894231209275024, 75.32525593107522, 103.50465408857391, 70.88228906086842, 137.05949527348008, -21.391578919413643, 17.452993778671118, -74.28015412841638, 161.8886862131715, -160.22677563780098, -130.01390552967283, 85.50199855139748, 128.38596640835615, -121.59232818847823, -33.20993764780209, 74.55743334328132, 66.42200841935036, 82.85731788823723, 144.73661805631355, 125.67758034765399, 14.98868430408663, -69.03663928605823, -51.988527513804115, -79.77940481800411, -116.19380224281828, -107.42722168981058, -35.69134681905849, 174.75441178526478, -101.92161273740993, -130.88909995796539, 69.22123191609907, 76.78213018978849, 51.47439759740991, -10.928159162012287, -84.58366291022344, -113.75342569786349, -169.11414397431022, -103.75633348741363, -169.24750566192068, 75.04831624649383, 156.12155513976924, 85.12738009422688, 160.28040509120999, -102.94619553740628, -164.31189394127335, -153.88757953386914, 27.063120984621424, -126.35598743623358, -87.20854517041057, -42.76163204693567, 28.14104632588827, -60.247899156709586, -76.29207556468022, 111.01831594824331, 3.7201428480367524, 13.816256693073122, 34.3725569193341, -86.50502117559476, -151.28560153052604, -164.24691915223192, 53.76348903229284, 8.681909644564268, -2.0861744162043423, 154.23769698066698, 149.64979409118288, -158.41567294084862, 148.18573741172742, 177.13762039147758, -166.49804400152183, -59.899376429272145, -69.41443913578352, -84.7464851555821, -128.234180608354, -117.05687221394788, -84.90710901560122, 179.28215149464526, 136.89005585002676, 73.50671399227849, 76.67752052907939, 60.36835961106027, 56.74038805160074, 166.0830798477666, -104.89704135120023, -141.35428443304292, -138.8515842919307, -145.823381488852, 60.15670847130603, -165.64091861835593, -166.26237995646107, -156.8844720489374, 127.4209843249037, 179.5225974398322, -118.64747350394946, -107.53591666959194, 83.12652344064755, 58.25050756657283, 127.95828104526579, -72.68488178548623, -32.9385602046413, -34.48484295221206, -118.19897384152911, -9.159861460160373, -1.9908690272106804, 103.28647111379468, -150.16725671533484, -116.7048000052059, -150.54030451455534, -143.47083256808807, -44.09451683879315, -143.654750090746, 123.78268889763535, 79.10268927262999, 80.2199996722576, 144.03595791080622, 175.23317832753972, 127.03318687319788, -156.29099534973514, 165.58681860738378, 111.32092075657337, -167.61296180695447, 177.09605248287616, 163.5363316581588, -30.883778883063563, -39.79292263260971, -18.586869222901267, -2.3755689451302335, 50.74953394094973, -88.70851302664174, -43.840541932610115, 155.7994445930218, -97.89185716035246, -37.01485713483075, -21.73304636487228, 143.9228065796252, 44.113716084197634, 51.813395808661134, 158.94340709510595, 5.776166563170778, 38.277033808929275, 54.00861681485472, 2.7495165090715616, 162.37373327110174, -149.65155764504877, -93.541125757921, 26.593331129604856, 51.083598367481216, -8.695570386692848, -175.30941717029904, 48.82394560004858, 61.833068258411295, 133.70266420091775, 62.03260725088454, 13.457131142113155, 37.356468170422374, -118.85456696685866, -179.8358274368663, -174.65255345609995, 105.30429364108664, 124.72552247214519, -172.02590182239177, -47.16748866302302, 80.01708528914783, 41.27087305290075, -87.47426159620247, -35.62391692534801, -42.57814140150857, -4.277118956842707, -101.91901828949577, 78.54214393850536, 80.94176306838557, 42.86335837716657, -4.905393454035079, 27.215224880766417, -97.99599959895087, 136.6592077635906, 137.9849247150967, 168.18066652707168, -137.31067142739977, -166.99669066127538, 163.7838737128681, 103.33146899300698, 92.07224115875105, 98.81318394011396, -55.890314881413616, 9.74255806186, 21.65883645732957, 25.865137050149276, -18.01117858600724, 23.746981559656945, -60.720679500608895, -86.93688915859549, -76.26178338790906, -133.2184146230326, -116.70514530033704, -124.06297782614816, 179.09750326916372, 164.86670746675134, 94.14267532171307, 149.8615369736314, -40.872645210521206, -48.87181798308624, -65.78932417679817, -150.59877319687203, -134.57577775971433, -86.15251143714788, -36.094323071721426, -25.117665174943763, -145.98243138627328, 91.36042392004097, 128.2891444595933, -171.58657183653511, -42.946851204696095, 40.22413973349145, 50.30939555866, 164.47408981773788, -117.63853371034936, -98.74009533091092, -130.92984057621226, -111.9078367767606, -70.48311140156457, 8.171283920611742, 73.09258450841943, 23.764641504616577, 67.20280668610175, 64.44182801361937, 9.387704000821607, 61.806845496539665, 98.88335535213105, 106.5507754149798, -8.452707276548043, 12.632978935407408, -114.01290845602558, -144.76304466637393, 26.692329951490873, -10.19908764398328, -54.54207719489448, -29.062527817579916, -49.52076791136569, -0.8287088438106212, -125.31960042860291, -82.91310197451543, -118.81133647501092, -171.46977649088888, 59.53118759400904, 58.89102015259415]}
  out "mag":cluster{"f0":dbl, "df":dbl, "magnitude":dbl[]}(graph)={"f0"=0.0, "df"=50.000000010186355, "magnitude"=[20.71924545043544, 23.301417028438195, 46.48569300062094, 32.68378710196127, 43.943351739114014, 38.149527232388905, 27.673425990177314, 35.17196325956325, 39.11669513760404, 28.183128702371853, 33.576052414237154, 31.24112685830844, 32.50966403781237, 35.7318815272326, 32.686807531319204, 36.25544918964384, 32.309812064251645, 17.496911132966446, 33.02559217265157, -2.0446502059566813, -2.0476129922073962, -2.0488902190055356, 21.88319158385941, 36.640486340902015, 33.3243255955274, 38.58078208701419, 35.82257182386253, 34.076307693075194, 36.02041459313822, 34.860143251540734, 26.17866054033483, 29.26292193790641, 38.62756895423501, 29.038153869144168, 25.025991258465123, 34.795598418617175, 34.159602360655725, 16.617320707304916, 25.95105830398628, 53.481288792711396, 59.74250116891575, 52.587202605851324, 25.352905236607953, 10.756657175584813, 26.602134177210726, 23.18255928152309, 27.161686421335073, 25.033803535627705, 1.2990173434335195, 20.45640572896321, 17.574046652411123, 21.090886189920013, 24.615968352810825, 20.524064027225393, 23.015214514927983, 24.188177432785327, 26.764733468460204, 22.08929098838015, 32.20500847452072, 37.71393587146687, 36.923602274391, 32.680853259831146, 24.336974304633195, 28.79472036507456, 28.269567955931137, 25.419700503767334, 24.208978046369836, 20.22907710994328, 17.93453077445198, 0.23157394622378938, 22.93715015969451, 25.67132178619326, 25.458268856201677, 23.745857906720907, 20.243404415239475, 20.790654583231365, 20.376482133221188, 23.018811580986696, 12.400370283027403, 18.057299389472295, 2.4847257487093937, 16.82183782101146, 26.446067076019478, 31.323396940457098, 20.046215450979673, 20.634460044799944, 28.22674606861576, 31.64565047389283, 12.747435171982769, 17.324563103122824, 17.203795291393014, 23.794659622967032, 24.776251043377467, 28.570086587388243, 22.136203664193932, 20.475349425419182, 17.54056693082008, 24.39986337203561, 17.494073122758248, 21.396754265344743, 32.42776382145958, 19.847815838956254, 13.735369300480711, 16.324927194270757, 21.165783133941794, 18.699181540519273, 20.355419114482164, 16.77830219633943, 24.6012152274944, 17.28485857434062, 14.816262050425465, 16.70786388703106, 21.89939618726646, 19.04229165429274, 21.04306455628741, 18.111856557541056, 17.003009277590603, 18.396891751724173, 14.707355834758067, 5.276740020785024, 11.836534018816494, 13.538681236452458, 13.194094270954137, 24.186635344453823, 24.052887821257517, 23.49573119810408, 18.629311357565857, 15.859296229244906, 17.770725714620212, 13.5511966424691, 15.493202733928078, 21.63028056380798, 20.297208901132784, 20.328322773254754, 24.555998344240734, 16.79088845019, 25.303583501920134, 23.709321849777943, 10.824003232485648, 25.44264864536367, 20.841414465203773, 22.26289650574969, 23.285597059013774, 17.960744365357208, 14.069184193228303, 17.4531094899965, 23.226668635740587, 22.074937009686614, 17.352244570245713, 1.6854631749952433, 15.930487728275367, 13.28101464402427, 21.50401250762766, 23.1545152113883, 26.248412092945912, 25.92165679430753, 16.378764388251845, 10.675158392492534, 1.1547083275469778, 17.828571865889078, 17.324135718952245, 17.241216142941866, 4.111200256867772, 21.31700395878148, 19.6136662838602, 23.554859700444652, 21.000185046392534, 20.639743576972776, 19.999863725683674, 15.879058145908756, 15.106503547565142, 19.59173549378839, 10.233771599734776, 12.459515705942168, 17.54842313324889, 15.32106381183941, 15.350945222762721, 17.754916666173482, 19.45647851293987, 16.284852154257948, 20.564834487220573, 23.14266400339218, 11.341447047613695, 19.330929746393394, 22.03706001782323, 15.769614087824982, 14.882468860136708, 20.402317527563465, 16.60248265505008, 14.535372622475254, 20.64807842946399, 21.28829984490173, 17.645774545872996, 25.482881094907384, 25.946540571243247, 19.854181092664756, 16.93824954557305, 23.62911955728679, 25.559729255801756, 4.387111308329986, 11.108960947180657, 14.020516531289076, 15.116466612872655, 14.07415154949582, 14.89214315538911, 22.48083685083936, 25.066481976408408, 14.70185632688828, 11.1987857200788, 14.493093984676841, 19.540959467050875, 24.740079499744944, 19.93311596201238, 20.05329763913651, 20.787429427098665, 10.88529239516637, 18.850712897552388, 18.448013408724993, 18.040627594063817, 22.030035105335948, 21.486383584389642, 13.606045305783933, 15.720071859868579, 15.219157882338417, 15.87816943841341, 18.825360936470645, 17.013657476566816, 19.068128898713073, 14.731095314474356, 11.559764635789232, 13.386393835385629, 12.246613616149126, 16.970050336142897, -0.41731169575055344, 7.81140962307158, 14.293701607222282, 20.41565877466484, 8.774853684949326, 4.729968256528921, 14.475503723270162, 13.076096827129156, 17.762720485911775, 9.838752792591322, 26.84154378660269, 14.623589706634144, 3.3000979154380805, 8.49496154117514, 16.031827201697862, 18.943544283973768, 14.152019180696971, 14.418768815329823, 13.875455644017965, 12.987696423439113, 23.362266623408317, 11.166817580095715, 9.666585212264344, 6.535600408893188, 12.099927365630634, 10.108284788728806, 4.866170251209895, 19.37358797180679, 15.653747626191784, 3.479281986840403, 6.444905479886502, 12.773112427595194, 15.68147726464108, 15.41806123204914, 16.105145232156374, 20.38236382958502, 0.7646408458412031, 14.36739801098012, 10.496184825922235, 9.017567417438658, 12.651662042471399, 18.304574878492662, 19.100580902248858, 19.100066742739582, 11.673511756228244, -9.353105825244821, 13.708207691996904, 10.985056327997523, 9.829578901343789, 1.5728385508916067, 14.713159990223328, 13.548978520329158, 5.734077674836467, 13.358307690872682, 19.091348838993362, 20.115692751729796, 15.102853137571557, 17.856859325142132, 14.217144713671793, 6.205672116066955, 16.456205027662524, 16.566471713937258, 18.660145129214925, 10.526925897761998, 19.403549250766897, 13.532049793290206, 18.752051084298532, 9.075233424273083, 7.054210211966582, 12.74299323632401, 16.52942281690719, 9.435755968151197, 11.613534918038624, 21.001935438991488, 16.301835149622992, 2.6512105089801556, 8.172146005421322, 6.198265135072829, 14.681350373799924, 13.545906350276617, 8.674618273527733, 2.3661118192208477, 12.234986030948283, 18.682384515862083, 20.824853058841466, 17.509316856811534, 14.430495084722885, 15.128051551611797, 9.407725920118082, 18.761720914897275, 13.659466149578547, 15.043776510991332, 0.9031895752087842, 9.025940716514528, 17.387685043316235, 19.44186773046323, 18.301262977585118, 18.58103529879071, 15.145850642980767, 13.214740411293576, 12.65356604563255, 15.25088392826699, 13.990028568843902, 3.2329273328138863, 8.598255906826857, 15.58401193451958, 12.532085713538878, -3.1303968418160726, 7.492067214177043, 16.539724941678898, 18.436155631440577, 17.363133079091398, 7.6426132760038445, 23.58053914092114, 19.623925825647103, 14.033804344994142, 11.091043783172998, 5.382244766122652, -3.172337842223225, 12.559313285137168, 10.84643221268113, 9.992473277303215, 5.064090670352449, 11.890773878598146, 12.458259260298206, 13.558865937312312, 11.988963639774251, 15.828594813781187, 13.395615700461772, 12.44792766368957, 6.360303015077631, 11.741447091989372, 0.7787568785060284, 16.17847446804395, 12.61895967243532, 11.365467062027598, 10.682861562426037, -5.553753068147867, 21.25101820644464, 18.310853138704413, 15.04312611430176, 14.658028009872513, 12.252462062506824, 17.9815221512364, 0.334497087498439, 8.733243562762185, 10.359883604209472, 17.017657129292587, 15.234287204073045, 14.123830540676117, 5.993308397106537, 1.0519723355984683, 4.997046476689725, 13.443166496951553, 15.17007841454691, -9.825032577594218, 16.66485767780815, 13.12213216565448, 9.568055228049115, 9.938125262226798, 11.992534439515472, 10.444073068476152, 8.292478602746362, 9.738310765840156, 10.557625040996424, 17.513347423343706, 14.145467801461704, 17.449198794780358, 10.231022107452588, 10.508125461028243, 15.945651504108708, 16.53553308330534, 7.85442894532393, 11.19177433977737, 8.659352390983052, 8.136956765649186, 10.769823592152072, 15.470229876357365, 11.628380175474504, 15.564012373090995, 16.126088544274072, 14.721364780205114, 1.04690625521779, 13.26456387340883, 18.517912592857865, 21.080359025380986, 19.794200071759363, 26.31179324971169, 20.85224199435716, 8.92990771285587, 10.715652528589919, 18.34627480408399, 16.424714539257227, 11.887796557372237, 9.49393389807242, 1.3277442845006446, 10.413626953460815, 7.776240541029781, 11.797200811513346, 5.35259077066908, 0.2262551224669268, 8.785384052598136, 9.450792605294636, 14.985673996647824, 11.903559879870134, -0.023144739636458796, 25.48677484294913, 30.801715985404083, 28.269086865532792, 9.508758586326936, -0.8495350935174284, 13.003123411126541, 13.259809566221088, 8.040981820812874, 2.426883944113129, 7.534151558099545, 8.230878728377007, 4.202203904723724, 9.231698426345387, 7.22735118250257, -2.967380931900563, 7.366766594429382, 10.368718398691357, 7.661450351807312, 14.022609626217239, 15.859272736164172, -3.8406268353829893, 0.48668641380033084, 8.218093316812329, 10.948411759015436, 2.9318225506494535, 2.536137132003563, -2.5265384526782637, -4.334518598690966, 10.101055185043148, 6.703731287789495, 6.6092614688106535, -6.717599535907043, 1.5874235974711497, 3.3655883362599432, 13.146564965364071, 3.423823965399203, 9.734347189142351, 6.2873431561148525, 10.674693668878225, 16.519603153766464, 19.604859728006797, 14.818368952011047, 12.742282611506763, 11.445918408137638, 15.072837651508625, 19.027187000040666, 10.852101658566562, 16.436749307154916, 14.551801714249326, 5.209856951347258, -2.055696462033007, 2.927006791898557, 6.099205308347036, 7.7359241886303245, 7.465288073109893, -6.523128666593786, 5.932538910062545, 0.7926998438649853, 5.486289174607329, 8.476944023900899, 12.696820079362013]}
  out "coherence":cluster{"f0":dbl, "df":dbl, "magnitude":dbl[]}(graph)={"f0"=0.0, "df"=50.000000010186355, "magnitude"=[0.9339546081175591, 0.8316339696569259, 0.3979384834199573, 0.11616313163418912, 0.35134026021484166, 0.571806665372829, 0.19804891560115556, 0.36733139100855217, 0.4132068186111416, 0.087602261043365, 0.5605797142709444, 0.33003991023269214, 0.586505889936099, 0.34641699755550337, 0.48334534514056154, 0.6700234790395019, 0.13113743366168204, 0.020225099774404034, 0.22862611076786366, 0.9999998001240847, 0.9999999374706827, 0.9999995823224481, 0.04004271146082056, 0.5215444217359061, 0.11900070962063955, 0.17584087412997365, 0.27394414106228016, 0.3604433106808488, 0.8277297567511068, 0.791797082276291, 0.35462033910477797, 0.20608816928605145, 0.44858121888901037, 0.7070927317399994, 0.16272958415442784, 0.44509192998073377, 0.558043476160264, 0.006428403008854959, 0.2826924903324115, 0.6298234904862126, 0.42405524652879506, 0.2396595114940291, 0.16670116612993022, 0.010555284691495302, 0.23885422882997814, 0.16282807288871484, 0.3563781598892667, 0.2690828876990791, 0.001655227194252132, 0.11966757796735546, 0.07869182772112611, 0.15902435377310867, 0.6071462248819841, 0.27667158028059463, 0.7753344161108123, 0.4129194926012443, 0.5986744660194896, 0.2331668548903566, 0.7081531890419464, 0.5996956123703404, 0.8184709970443875, 0.4672023182018119, 0.49850542665222675, 0.7576073865410411, 0.665216612149718, 0.6276454930794088, 0.16985017495537924, 0.13771121831080907, 0.12926566940686166, 0.00760489657477854, 0.3956388334514201, 0.4939057805554319, 0.3238136074533217, 0.2236133871553565, 0.2097691290417539, 0.08854945720810278, 0.020957006170717284, 0.28981405407738825, 0.10399277056662638, 0.3807201744971528, 0.03332416494605055, 0.2568412394517988, 0.6333785063530032, 0.2624445676135391, 0.09335668228056548, 0.23714896519279707, 0.34369410320233906, 0.49788920800636977, 0.07009078784946045, 0.215423362231197, 0.14885636430005322, 0.44415002871188264, 0.4714708321013261, 0.5207225335693634, 0.2595709518548846, 0.5071546456094274, 0.21702784926213292, 0.7385431651152617, 0.4423933150020991, 0.14870394635942158, 0.507265848148348, 0.03680676388622598, 0.15051077307962954, 0.2649765277839596, 0.5173562743102679, 0.32747509903756467, 0.33628547814378784, 0.08430237591678327, 0.3605533738772842, 0.1584994637262605, 0.16359446221928722, 0.12393522215658988, 0.41470192140080875, 0.13371087418132316, 0.4484505029354363, 0.1721475628422095, 0.10022590563866418, 0.08024839731639388, 0.08554584106163408, 0.008107279887194462, 0.10544237522838043, 0.2784857785976977, 0.07017826295587644, 0.16056257003930366, 0.15419181607433372, 0.2877098776154182, 0.163442183316755, 0.16866813044619466, 0.11174527319363774, 0.1994281679336881, 0.19316297922200276, 0.5825409511188835, 0.38497291841433096, 0.3429350831694888, 0.31743026681036196, 0.1881533212852768, 0.6722752050876489, 0.35425285869699996, 0.0463535180931857, 0.43697873757831046, 0.10823762708083572, 0.24413091509073181, 0.17534841500772969, 0.3415857951797028, 0.16512176167512488, 0.2722161723079078, 0.7931978632008856, 0.2570064611227622, 0.26238854730577665, 0.00766650380981299, 0.08262528434742072, 0.08093904720633706, 0.47008036450474033, 0.5903441480640057, 0.49509728986187496, 0.4635487056852859, 0.19632136276619136, 0.04632050549252163, 0.002589331972438263, 0.24128159960189194, 0.5154471728742781, 0.3050962845293827, 0.003405404206269003, 0.5151618719647031, 0.39100448080146716, 0.5566508278349991, 0.6635163593074528, 0.5323521864522771, 0.44062244558676855, 0.15490886328203413, 0.14770940094156365, 0.35922106929086084, 0.03749545099781841, 0.052345978759194084, 0.33362371728107804, 0.32116059726938906, 0.17321224379690156, 0.30992206137207684, 0.3854072977944601, 0.20267202036949336, 0.4158074730245596, 0.5030826429389214, 0.16458873786850514, 0.35192080860941, 0.509651725727319, 0.25252895454602753, 0.10414136318849312, 0.21906161820774944, 0.08986526365223506, 0.17886160642420354, 0.37700116740082207, 0.4341575769409633, 0.2650805917681961, 0.4421881328779682, 0.603738378921592, 0.6112540789927805, 0.5116014432687817, 0.267060420686285, 0.6609766618985682, 0.013972513874619372, 0.1973281361118622, 0.09400960018039047, 0.187017884611303, 0.6576043675046809, 0.47610274175367373, 0.4125286646512166, 0.30560803621381916, 0.12651756208861364, 0.13797211189687555, 0.15761232904864847, 0.27539236389795857, 0.7136317787318104, 0.3188403847964556, 0.5103945180645831, 0.3284510669422444, 0.11329136806112355, 0.3829165741928596, 0.18960115834254032, 0.16437635196288908, 0.6471560003038982, 0.5049162626321875, 0.14666216397727125, 0.2425427616704399, 0.10633721918761595, 0.2488907753936048, 0.21772971030687904, 0.2149776182438685, 0.34370525577806776, 0.41612158995246223, 0.07175551908111712, 0.17937688583714623, 0.21340721972117213, 0.40676507338655543, 0.013141775731946855, 0.13967363325227908, 0.12971342444971437, 0.2776093109035508, 0.1394062972068387, 0.0489306167042301, 0.20346997446205653, 0.5343022854739391, 0.3267736969604767, 0.05229656160964828, 0.23154300362968558, 0.043438340919333976, 0.061155510142968265, 0.20797461403758946, 0.4928116656204711, 0.44686474762579553, 0.10244817233270588, 0.11066568452349858, 0.23376568592710983, 0.07874186106747742, 0.6001871395141181, 0.21123594407657062, 0.30633732552337173, 0.3481596730344442, 0.4101311417905852, 0.14275023942765908, 0.04127889391876968, 0.28224781761550904, 0.4444122770293498, 0.0814375774473262, 0.05818801359488662, 0.0874387137912153, 0.157687182538937, 0.4393913315368055, 0.17335841822499234, 0.3730823310314625, 0.0057714341968473715, 0.30500015980899337, 0.18077343718796599, 0.10931787410397223, 0.2796335468707271, 0.5380934961923053, 0.33357188227824236, 0.3138868493363831, 0.20428494805518121, 0.0014002237257722398, 0.4728888741277729, 0.36077642353757866, 0.0711685127243101, 0.01570090945642336, 0.40356064942976133, 0.3748100509347576, 0.03477437268687251, 0.05977854638904302, 0.2706113778656578, 0.5930002053340881, 0.47649351958603253, 0.6801449480262717, 0.37601447382310504, 0.017617980273724528, 0.0762079399156292, 0.35118616631472266, 0.3330822369289068, 0.11750167477118988, 0.5269396944819398, 0.33141716902245133, 0.4711401613621411, 0.11691521829910183, 0.03273819175188156, 0.1203733217446241, 0.6768602112556984, 0.49066362840702876, 0.23069585969130144, 0.8290138805485532, 0.256096317038154, 0.02582396910258949, 0.24617967772340563, 0.21543638336504264, 0.4636259380299981, 0.3975493866057751, 0.23296236155525804, 0.04823930562463316, 0.1882859685974336, 0.5163736622966277, 0.47321077477220647, 0.2946126078922972, 0.2167098022612296, 0.5784110218223546, 0.22556115759614523, 0.2698812796856335, 0.14296268186197436, 0.4253918510072807, 0.006687497106601638, 0.05718936608023608, 0.5038696263707731, 0.7250621166924622, 0.15014635578798632, 0.26089414251892684, 0.4638822878796963, 0.4374970260638938, 0.3480515283266393, 0.45059385951724074, 0.338587518900865, 0.01860519055290668, 0.05997273415963626, 0.21297317644364483, 0.6529660048319023, 0.26368982895424303, 0.40937472752381315, 0.3354069848135074, 0.2279593665589126, 0.11267986478339324, 0.010698717133293775, 0.5220410335323572, 0.4965881234923157, 0.13210636722939714, 0.19263632537451292, 0.11607531010420828, 0.010024843022708502, 0.15167971254236684, 0.3110198657353013, 0.29347698595136523, 0.1414340677906298, 0.16043505529994348, 0.26040589049005686, 0.544531996472485, 0.6084819345209863, 0.7424633313191171, 0.35232758580789497, 0.28434311851028743, 0.21594330895766353, 0.22685738302614736, 0.14160938703807768, 0.6358884405427145, 0.3873779004135953, 0.23515196083035453, 0.2432127906842056, 0.010872312252655367, 0.6575000615065131, 0.3315868940571207, 0.3764478188024479, 0.6001248819192951, 0.09003662763374858, 0.361991426030318, 0.031521163651871534, 0.4402453402809462, 0.25773093670557085, 0.5483818620037105, 0.2299246901584136, 0.42800310610553444, 0.13539727373390897, 0.059422143332086536, 0.27244131209278655, 0.5925129308981769, 0.5441278386269333, 0.002889775238752289, 0.35796615892061384, 0.1693046120139347, 0.21254624819612392, 0.2655846021537521, 0.14040877688912426, 0.06695681261615541, 0.3369382775686377, 0.41836842437118354, 0.24849567366463837, 0.25231208612086686, 0.30791121457981774, 0.7472599886049438, 0.12404628805263972, 0.11326623799188601, 0.1836170897092732, 0.3664455227985015, 0.16077797442240127, 0.48716562287490056, 0.30847405704825265, 0.26661012578685506, 0.06055435447149417, 0.5636412275914977, 0.12327710594704042, 0.24605172088870544, 0.42057786642928957, 0.6603240119667892, 0.06287386533942277, 0.5184975359643509, 0.7289165819372484, 0.45166985594110853, 0.5735521989060992, 0.7743545573459891, 0.16656079993393225, 0.14605865361080658, 0.3764426400025425, 0.5080887011701367, 0.15894002313527744, 0.17285607010877443, 0.3986843389797408, 0.02715779482167682, 0.44304600365547653, 0.5259932309355195, 0.5185081106503653, 0.13230024221434114, 0.04190059440430736, 0.21625089827096972, 0.16302060063225235, 0.5561766480939072, 0.6053202879664901, 0.11037676335199804, 0.6705540221992806, 0.8488565315360331, 0.4161746941809008, 0.34646559326825604, 0.004248292917352837, 0.17407167118160216, 0.35312458184031453, 0.3137961540190362, 0.026093413781326374, 0.23331101133965512, 0.33031813727876214, 0.2781650630114178, 0.5217178804798005, 0.16507378429845304, 0.05123396717708542, 0.33050425612516354, 0.16578666985160087, 0.09827321955536396, 0.36359325201961973, 0.47893957590326625, 0.20029333549338263, 0.8248943569048484, 0.6449709011336435, 0.14923080740932426, 0.09942912956647379, 0.1862931391074277, 0.01889584878553142, 0.01618386038762885, 0.49212055923423853, 0.26294740254916277, 0.24572531392388983, 0.021316867703167264, 0.03957454962851278, 0.026099725065342746, 0.31296659200233434, 0.06708040166640233, 0.1656086195063649, 0.10622077592194745, 0.18678047673359796, 0.338482527835264, 0.6061853082478812, 0.7518581476616196, 0.6481981955531527, 0.6090730654180362, 0.5218151424531249, 0.5448178152923564, 0.291512588420024, 0.5647362298292679, 0.3266886541711634, 0.1600006277752436, 0.11498375564782022, 0.20091930250798923, 0.6355458601242946, 0.6278115416780897, 0.2765545008906038, 0.008440376956111783, 0.11066133072009156, 0.0708167916592605, 0.18506953135714613, 0.23727410037169613, 0.48050133170697407]}
  in  "maximum harmonic":i32=-1
  in  "harmonics to visualize":i32[](array[numeric])=[-1]
  out "expected fundamental frequency [Hz]":dbl=1000.0 format="%.2f"
  out "actual maximum harmonic":i32=24
  out "THD":dbl=0.5084385378838435 format="%.2f"
  out "detected fund. freq. [Hz]":dbl=999.9796682823572 format="%.2f"
  out "fft":cluster{"f0":dbl, "df":dbl, "magnitude":dbl[]}(graph)={"f0"=0.0, "df"=50.000000010186355, "magnitude"=[-49.488795253665295, -50.627142477944105, -64.17200476260074, -74.90264444011959, -68.98003210303047, -71.57823336519711, -75.29280899119628, -74.03736014882409, -83.59387272012968, -87.69793259864184, -81.30730791822687, -79.1439673441838, -80.37430304528823, -80.77752900265585, -78.85680852728561, -77.52180632515946, -81.80568159659686, -86.85447954288179, -82.73595072844037, -15.442515877025505, -9.426202721724628, -15.450180576756946, -82.7033211491468, -86.18120305445623, -81.94713324804508, -76.04828339242734, -75.9420369660573, -81.5033205016084, -80.43403918559333, -78.00318085347891, -84.8754827086739, -80.57673837416462, -78.12955710285547, -83.88507570306372, -84.45538274522906, -81.56127381114992, -84.19495532321139, -85.68210095194821, -88.36167803616789, -61.197352641957146, -55.41922649813354, -61.475669116059414, -99.13241804807855, -92.91323760923004, -89.93833722188, -100.88410909011257, -86.45442096188093, -87.59385741692797, -92.62333859969911, -94.83722848183314, -96.07274848580091, -93.1563450802823, -91.98038573787534, -93.71816741472475, -92.25072357632993, -90.23103041146976, -90.90876511052019, -95.78879673637908, -88.0395819709078, -78.26796829928557, -74.6116615260879, -80.56268815768118, -96.96303727554222, -96.52939135028336, -92.29492499552263, -92.17938298508417, -93.10385073760722, -98.6638113525329, -100.86800213804912, -107.40967076417672, -93.49717255833077, -89.85039064586377, -87.45164175702483, -91.68439894856834, -103.73743247619244, -95.54442177255213, -96.98395721600563, -103.56560876089318, -113.51510692956734, -99.26070077945893, -105.7904532939472, -100.03044190330655, -92.21946185088859, -93.84822513205029, -105.66840988334648, -92.11560730924467, -86.63326947720486, -88.61937130019749, -98.08607876112853, -103.06162710611191, -95.83082395970703, -92.67364769254661, -96.97267275940573, -92.9455208091102, -94.32448894337656, -103.38771268745155, -100.68182315540415, -93.55409501895566, -95.83246026029718, -90.74845106254875, -84.36975503757643, -90.06821687231286, -101.72686802136406, -110.53939915087972, -99.46700054596701, -95.20387226508578, -93.35221547186768, -95.9062813405261, -94.6495334050897, -100.45434825363657, -99.3031200015457, -99.05327540619352, -97.06178557333571, -102.99181173858345, -97.45258904529636, -103.63189199809229, -107.80794672120714, -107.21966071268234, -106.17059160111161, -97.85751695939672, -96.25589039093813, -100.64041322642089, -106.26044470674144, -97.29677276563172, -95.09070255228323, -90.51570944006332, -91.84379079964745, -96.59032256242625, -100.45177841179866, -114.68835421064158, -111.21396871397872, -101.33001076847557, -106.15979470234439, -95.88781383042902, -94.59569299244139, -102.87620744171852, -94.1970171653292, -93.6632552068984, -95.37915612684456, -89.41710157230878, -89.62792213905773, -94.43798798947554, -106.77168498471025, -99.4710420835701, -94.62696312870929, -91.97084485673635, -96.04150820792569, -94.72650307508883, -103.3124741153371, -107.8283740926623, -103.53121330007758, -104.13979040948018, -100.91135543883485, -96.87552094063324, -89.97943488668973, -91.65705932159992, -101.02313693197408, -102.30820611527614, -96.53980712327117, -98.08163808872898, -104.891830426784, -107.06467646799862, -101.38337020728278, -98.15342018797033, -95.58573239014814, -93.11157828932645, -97.81365617245459, -102.82617401019905, -98.01911856678053, -100.92566378177406, -108.17344340432298, -98.04350102272521, -100.53621379844068, -97.71239948196796, -96.00460979639516, -101.03417045655493, -97.72762565204806, -98.61772549696633, -100.34554824519091, -100.88047810507966, -98.85061238027787, -98.30852425501753, -103.38757995244629, -99.06398258670222, -98.64078893684139, -102.51506714008752, -103.12473327916842, -96.1376818305572, -92.88351897497344, -99.95123516907915, -96.89090477653066, -103.22696178711234, -97.73483825869954, -91.3076509729564, -92.11140160896963, -95.25602889878064, -101.31358236451489, -97.43809623420691, -94.03370986815409, -98.10343047492381, -99.90613779738123, -101.54657082458483, -106.52271417821422, -106.87880011449927, -100.77727220909253, -97.90635599856431, -95.33692079897367, -100.84583706022853, -102.99839662919373, -102.00187801615373, -98.85619056653121, -95.86203240082423, -96.03522894028215, -100.17619294243651, -101.80194218273698, -106.2108468436563, -104.01686520592403, -98.62474555502475, -96.83482205098773, -108.52337747302776, -97.67636542262053, -96.47229997309189, -99.53982807439813, -105.48669245125679, -103.82231573380666, -102.03945686600397, -118.17072553274647, -101.56087764440184, -102.12588207396402, -95.13433162420809, -100.90800681396249, -102.54559156349254, -98.3611326406318, -103.80924738008915, -106.79732102574427, -101.95918283411686, -103.94029674793542, -103.35461256420427, -110.9609119013112, -105.82536006200803, -113.81266617612675, -99.35596024061616, -110.32932734991483, -95.82860843788305, -97.07514351814291, -109.43354731640954, -107.3646912741749, -101.77832770845946, -101.70801212308103, -101.73292359030438, -96.86441145675275, -104.3154668714775, -98.80626739508517, -100.63741596432308, -101.01697701941492, -102.03634025045139, -107.36446456004501, -109.57920182099421, -111.65524303692854, -104.37562364049357, -98.79471578647994, -106.26943945762252, -109.45364154451538, -110.89199369381785, -118.52147878906808, -113.15044987985019, -105.9628787985668, -98.84454636419035, -98.16235091331846, -102.04618866435602, -107.19227607904566, -102.08203465166577, -103.74114857412292, -104.00922981266193, -97.85865038232265, -100.87940822215657, -100.01702177467484, -101.91580164910236, -104.99363489576086, -110.45525721965312, -110.52265260528458, -108.15437303215404, -116.2223935456526, -105.64487805436661, -108.68342755035683, -101.7666351753116, -99.03495652388749, -98.30468097063631, -97.92527829293037, -101.11033315396557, -100.29541819249621, -104.668681889644, -114.96674472709222, -102.20873205694286, -102.89953106104323, -106.67135472191282, -105.55691372078286, -95.89106251068009, -101.5665323471182, -100.9401536866153, -106.15874884487347, -111.49419472212357, -99.98403925555735, -96.83209673444858, -105.66710385232616, -105.77987572747018, -105.96460073011318, -105.63540052511215, -107.7913377280531, -106.71249278729071, -107.43921464655615, -102.54391474319851, -101.92313119313424, -102.36054622039354, -116.4188287655894, -105.2704103277651, -107.18581313805977, -110.01868123302108, -106.42865981969557, -97.9034782473023, -97.36507437246011, -106.03337533464567, -104.10709004569696, -103.42800411743187, -106.62941637998559, -107.91907894875713, -111.3921869949334, -102.91506618303313, -101.17219079356039, -101.1882445773982, -99.33954317730434, -105.93345010709213, -112.03864557590279, -104.10187763152095, -97.38690680539978, -99.22583009804967, -107.47071652682249, -106.70783972234489, -100.77492191669788, -101.82682608451488, -109.51600060080298, -117.15317970350647, -104.18687204589128, -96.36752546300634, -96.05776967950838, -98.80043380861648, -100.49332268387161, -99.30314268742305, -100.9706744641445, -108.23181196391117, -108.75025140286101, -107.76814411220008, -126.82930486462412, -133.1255093821169, -111.71714151331804, -110.09765264385649, -103.98307412295998, -114.84595040981759, -105.59315843444557, -102.27192459533995, -96.68183870174701, -100.50330593664455, -100.17678108311566, -110.10987021200906, -109.17166700424471, -112.30161357467118, -100.91627829630195, -101.84238957700086, -98.25428755155446, -97.93921350263335, -109.72358629781161, -102.23834646880321, -102.35901019887336, -109.39836876691488, -106.3572455544577, -101.34957160409618, -101.72039326889136, -105.30936567429121, -106.59210119315226, -108.57432094915393, -100.71983988224984, -102.5388111063985, -112.09207437132662, -113.91709132702636, -113.79289844404354, -121.9446788115588, -103.50741710900708, -102.05253528564833, -110.80040041990716, -102.44945076514111, -111.48340232772031, -125.2555467113875, -103.8720226467632, -101.63700900956455, -102.09092704232306, -113.49801670293598, -110.79534142157448, -104.65855732294028, -101.44322221209367, -106.37795949620944, -104.97136833004056, -105.17553703117072, -108.21134255992928, -100.66493542975353, -100.58832041297134, -106.84385039721212, -112.47917437286573, -112.57950782042117, -111.45615370145883, -106.91694474821212, -104.77875275871993, -101.78812793379072, -102.54458723586737, -103.35435460821218, -106.1221420107264, -109.79236545719574, -113.37536124974649, -102.06120269648258, -102.67560629184017, -101.46571635663243, -94.64698544028113, -101.86116186844613, -110.82993493510895, -105.73883082028675, -100.78254014352342, -102.55867925930124, -106.44553867302406, -107.47494516320717, -106.02541951488446, -110.79184158705154, -108.28855336561345, -105.72041660751117, -117.69651179539365, -117.1486159905792, -105.8120036360742, -105.8930575217255, -107.29607934473805, -106.93281203249073, -116.2717162977707, -94.57002067208295, -88.12081006268207, -94.70381117559586, -113.47970564744219, -111.7401283685608, -113.540583901378, -104.091622621751, -108.98402025990129, -108.63652162317025, -107.1708336143409, -111.15937455988788, -113.13178714408417, -109.31519733176356, -110.733157063207, -118.842569848165, -117.84291808621927, -107.72682331910897, -113.47779010817626, -104.3320052791971, -108.16153231864914, -110.94814250262081, -105.41096742290935, -101.26296624959936, -103.10652081924245, -108.35334238898314, -109.62724860454321, -108.83756198910719, -124.86894797808056, -105.60303476002632, -107.07312325079513, -120.55754367560777, -117.94297950098512, -107.93518245977023, -103.96442203203617, -106.68733378561723, -106.1342582703219, -108.50246667581374, -113.76564617495785, -104.86926619554382, -102.17416004857542, -102.40703850123809, -103.67810652546427, -104.79006949551291, -102.79559870429847, -101.36967516119456, -103.22006919849062, -110.9414908696807, -110.05293004940069, -106.79962984847124, -108.83060617039085, -122.36594013651107, -122.6151499988862, -114.79560361444337, -114.11638639654487, -118.32690344894674, -113.6961399255385, -111.67849160037204, -118.22210929693804, -116.38677597409247, -112.65664265527433, -112.50019329465812]}
  in  "dB On (T)":bool=TRUE
  out "coherence 2":dbl(graph)=999.9999374706828
  out "COH":dbl=999.9999374706828 format="%.10f"
  in  "stop":bool
  out "loop time(ms)":u32=19
  out "Coh_FR_Time Chart":cluster{dbl[], dbl[]}[](graph)
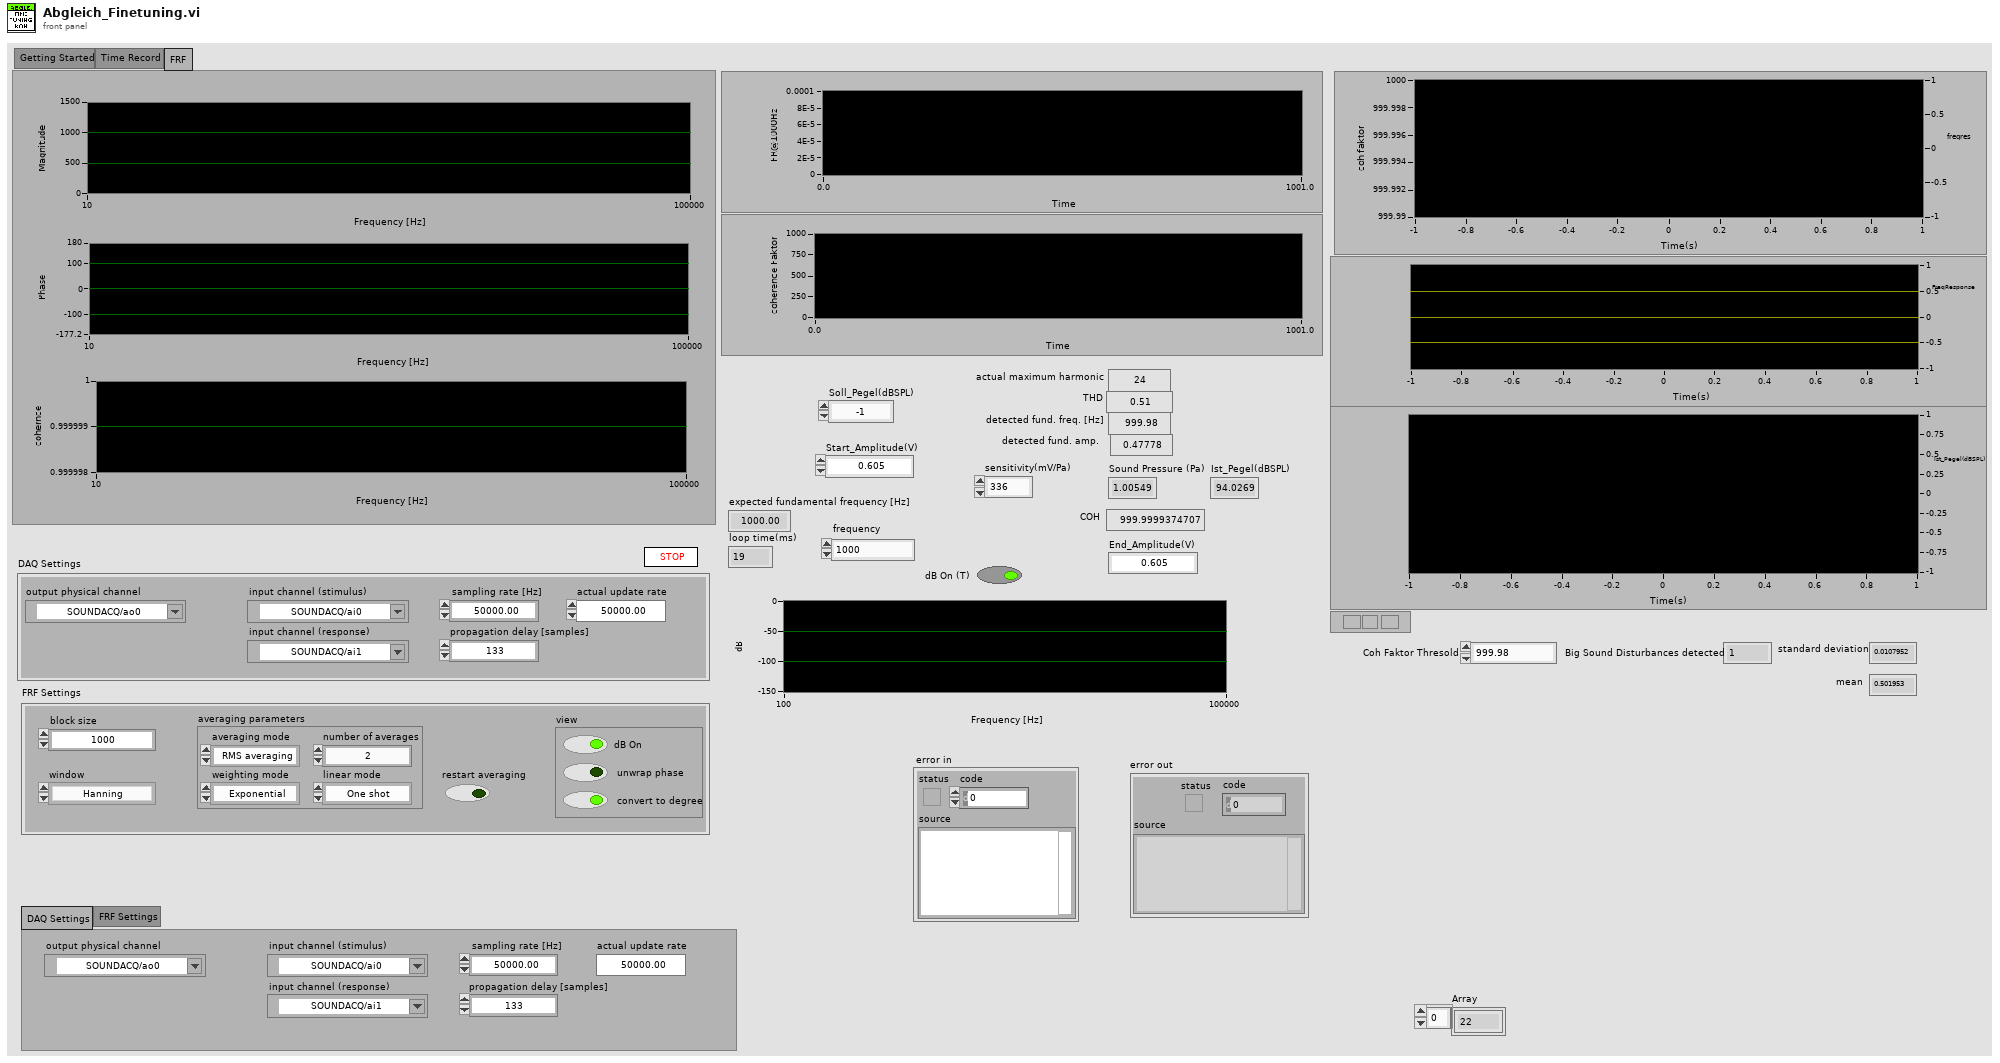
[diagram p1: front panel]
types:
  T1 = cluster{"sampling rate [Hz]":dbl, "actual update rate":dbl, "output physical channel":tag, "input channel (stimulus)":tag, "propagation delay [samples]":i32, "input channel (response)":tag}
  T2 = typedef "svc_Window [Dual FFT].ctl" = u32
  T3 = cluster{"window":T2, "block size":i32, "view":cluster{"dB On":bool, "unwrap phase":bool, "convert to degree":bool}, "averaging parameters":cluster{"averaging mode":enum16{"No averaging", "Vector averaging", "RMS averaging", "Peak hold"}, "weighting mode":enum16{"Linear", "Exponential"}, "number of averages":u32, "linear mode":enum16{"One shot", "Auto restart"}}, "restart averaging":bool}
  T4 = cluster{"averaging mode":enum16{"No averaging", "Vector averaging", "RMS averaging", "Peak hold"}, "weighting mode":enum16{"Linear", "Exponential"}, "number of averages":u32, "linear mode":enum16{"One shot", "Auto restart"}}
  T5 = cluster{"dB On":bool, "unwrap phase":bool, "convert to degree":bool}
  T6 = enum16{"uniform white noise", "Gaussian white noise", "periodic random noise", "Chirp"}
  T7 = cluster{"THD units":enum16{"dB", "linear ratio", "%"}, "harmonic component amplitude units":enum16{"EU rms", "EU peak", "EU peak-peak", "dB ref fund"}, "detected fundamental amplitude units":enum16{"EU rms", "EU peak", "EU peak-peak"}}
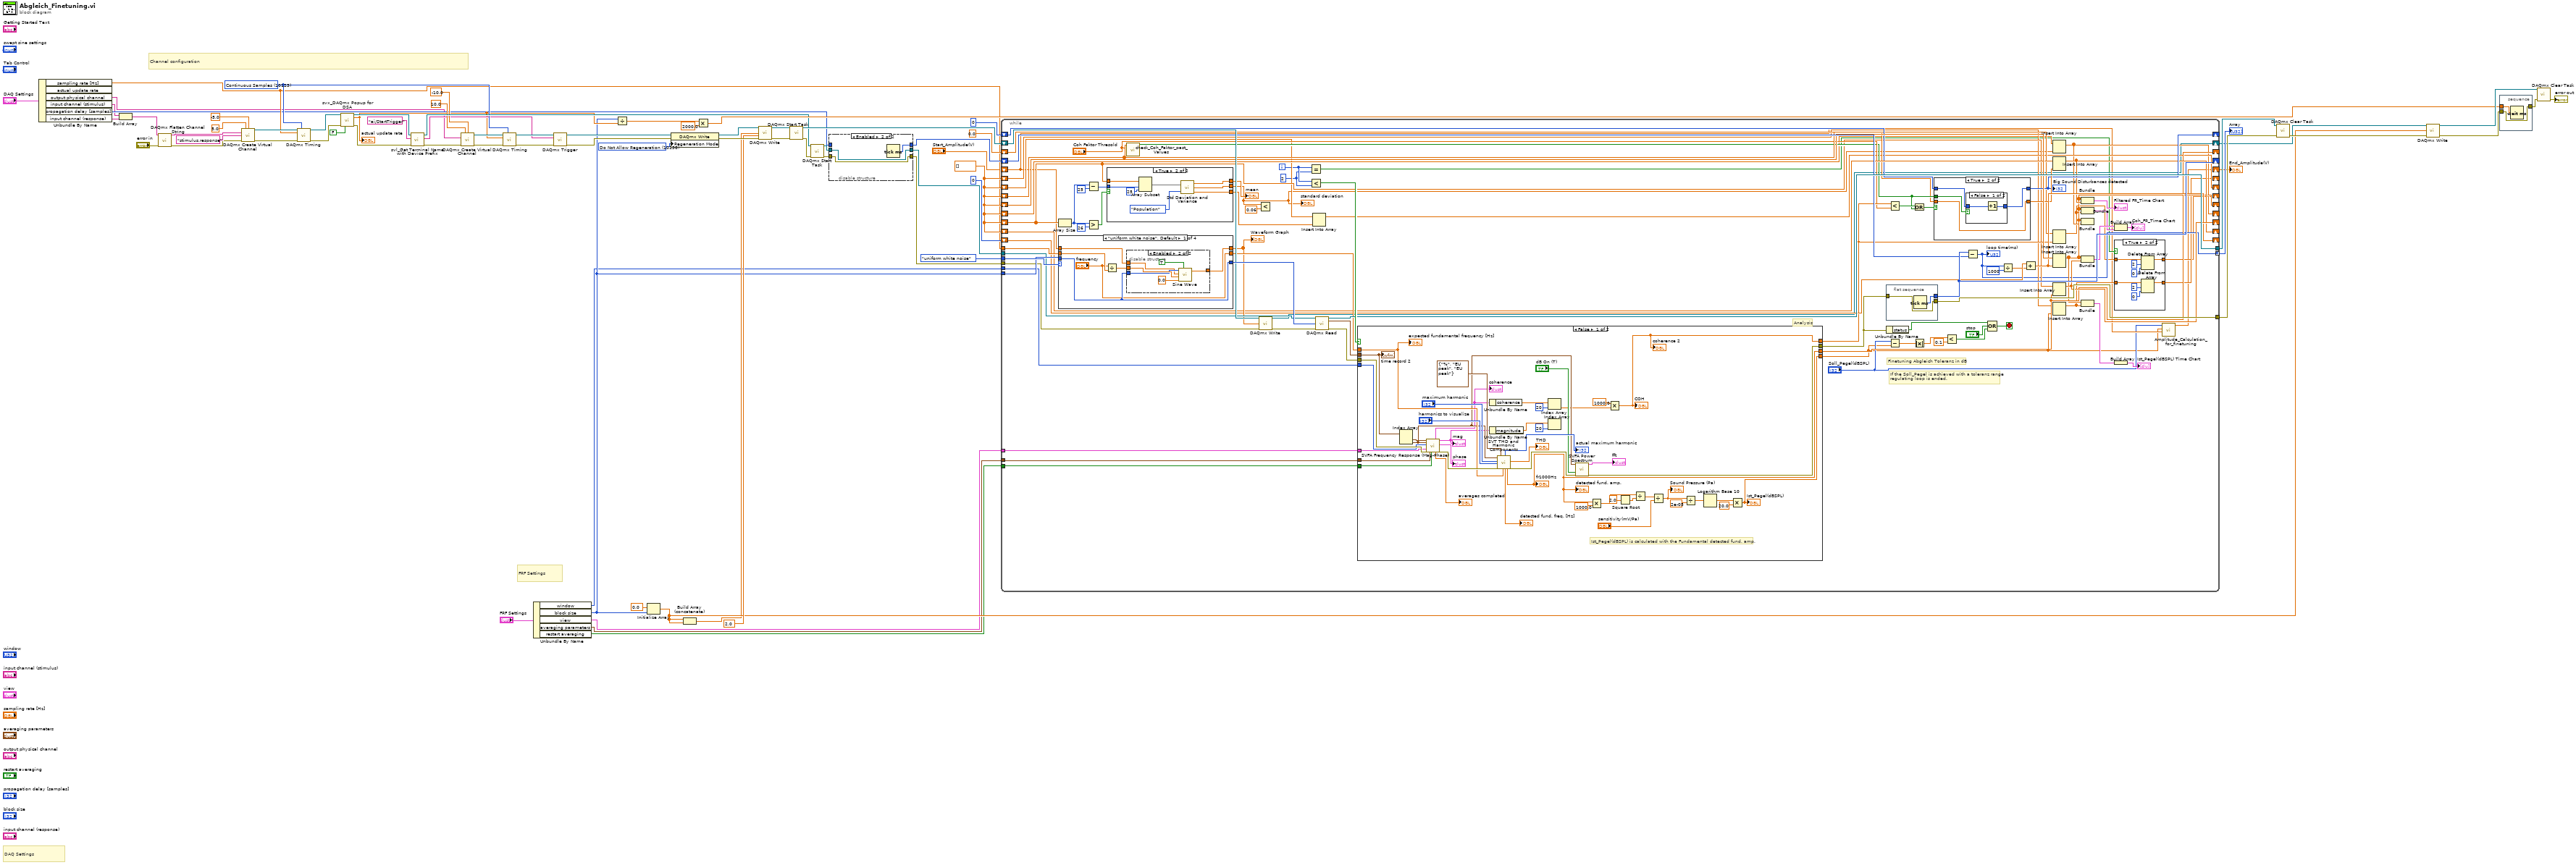
[diagram p0: block diagram]
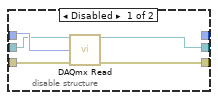
[diagram p2: hidden frame]
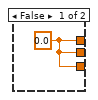
[diagram p4: hidden frame]
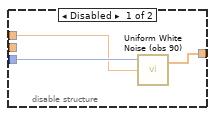
[diagram p7: hidden frame]
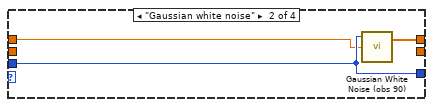
[diagram p8: hidden frame]
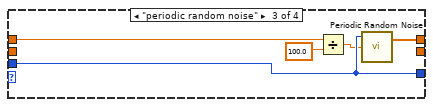
[diagram p9: hidden frame]
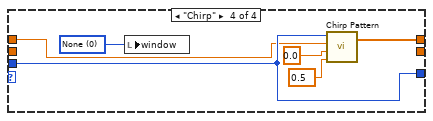
[diagram p10: hidden frame]
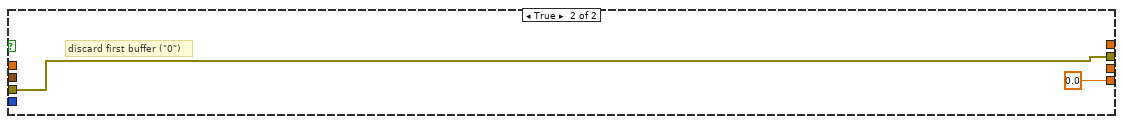
[diagram p11: hidden frame]
diagram:
  w22 = dbl[] []
  w63 = 10158 items=["Allow Regeneration"=10097, "Do Not Allow Regeneration"=10158] ("RegenMode")
  w32 = 10123 items=["Finite Samples"=10178, "Continuous Samples"=10123] ("sample mode")
  # "Channel configuration"
  # "FRF Settings"
  # "DAQ Settings"
  n1 = Unbundle By Name("DAQ Settings") -> ("sampling rate [Hz]"=w15:dbl, "output physical channel"=w12:tag, "input channel (stimulus)"=w11:tag, "propagation delay [samples]"=w14:i32, "input channel (response)"=w10:tag)  [unwired: 1 out]
  n2 = Build Array(w11, w10) -> (w27:tag[])
  n3 = call <vilib>:"DAQmx Flatten Channel String.vi"("names in"=w27, "error in"="error in") -> ("names out"=w26:string, "error out"=w1:errorcluster)  [unwired: 12 in]
  n4 = call-poly <vilib>:"DAQmx Create Virtual Channel.vi"("maximum value"=5.0, "minimum value"=-5.0, "physical channels"=w26, "name to assign"="stimulus,response", "error in"=w1) -> ("task out"=w44:refnum<k21>, "error out"=w43:errorcluster)  [unwired: 9 in]
  n5 = call-poly <vilib>:"DAQmx Timing.vi"("task/channels in"=w44, "sample mode"=w32, "rate"=w15, "error in"=w43) -> ("task out"=w30:refnum<k21>, "error out"=w29:errorcluster)  [unwired: 10 in]
  n6 = call <vilib>:"svx_DAQmx Popup for DSA.vi"("task in"=w30, "error in (no error)"=w29, "interactive configuration dialog"=FALSE) -> ("task out"=w39:refnum<k21>, "actual sample rate"=w28:dbl, "error out"=w38:errorcluster)  [unwired: 10 in]
  "actual update rate" <- w28
  n7 = call <vilib>:"svl_Get Terminal Name with Device Prefix.vi"("error in (no error)"=w38, "local terminal name"="ai/StartTrigger", "task/channels in"=w39) -> ("error out"=w42:errorcluster, "terminal name with device prefix"=w31:tag, "task out"=w41:refnum<k21>)  [unwired: 6 in]
  n8 = call-poly <vilib>:"DAQmx Create Virtual Channel.vi"("maximum value"=10.0, "minimum value"=-10.0, "physical channels"=w12, "error in"=w42) -> ("task out"=w73:refnum<k21>, "error out"=w72:errorcluster)  [unwired: 10 in]
  n9 = call-poly <vilib>:"DAQmx Timing.vi"("task/channels in"=w73, "sample mode"=w32, "rate"=w28, "error in"=w72) -> ("task out"=w71:refnum<k21>, "error out"=w70:errorcluster)  [unwired: 10 in]
  n10 = Unbundle By Name("FRF Settings") -> ("window"=w9:T2, "block size"=w13:i32, "view"=w8:T5, "averaging parameters"=w7:T4, "restart averaging"=w6:bool)
  n11 = call-poly <vilib>:"DAQmx Trigger.vi"("task/channels in"=w71, "source"=w31, "error in"=w70) -> ("task out"=w67:refnum<k21>, "error out"=w66:errorcluster)  [unwired: 11 in]
  n12 = Divide(x=w13, y=w28) -> (x/y=w50:dbl)
  n13 = Initialize Array(0.0 ("element"), w13) -> (w55:dbl[])
  n14 = property class="DAQmx Write"(reference=w67, error in=w66, "Regeneration Mode"=w63) -> (reference out=w65:refnum<k21>, error out=w64:errorcluster)
  n15 = Build Array (concatenate)(w55, w55) -> (w49:dbl[])
  n16 = Multiply(x=w50, y=2000.0) -> (x*y=w48:dbl)
  n17 = call-poly <vilib>:"DAQmx Write.vi"("task/channels in"=w65, "data"=w49, "timeout"=2.0 ("Wirite Timeout"), "error in"=w64) -> ("task out"=w69:refnum<k21>, "error out"=w68:errorcluster)  [unwired: 9 in, 1 out]
  n18 = call <vilib>:"DAQmx Start Task.vi"("task/channels in"=w69, "error in"=w68) -> ("task out"=w60:refnum<k21>, "error out"=w40:errorcluster)  [unwired: 12 in]
  n19 = call <vilib>:"DAQmx Start Task.vi"("task/channels in"=w41, "error in"=w40) -> ("task out"=w45:refnum<k21>, "error out"=w46:errorcluster)  [unwired: 12 in]
  n20 = disable-structure shown="Enabled" {
    disable-tunnel: w14 -> [w80 _]
    disable-tunnel: [w79 w83] -> w59
    disable-tunnel: [w78 w82] -> w58
    disable-tunnel: w46 -> [w77 w82]
    disable-tunnel: w45 -> [w76 w83]
    disable-tunnel: [_ w81] -> w19
    frame Disabled {
      n21 = call-poly <vilib>:"DAQmx Read.vi"("task/channels in"=w76, "number of samples per channel"=w80, "error in"=w77) -> ("task out"=w79:refnum<k21>, "error out"=w78:errorcluster)  [unwired: 10 in, 1 out]
    }
    frame Enabled {
      n22 = Tick Count (ms)() -> (millisecond timer value=w81:u32)
    }
  }
  n23 = while {
    tunnel: w13 -> [w164]
    tunnel: w58 -> [w155]
    tunnel: T6."uniform white noise" ("excitation") -> [w165]
    tunnel: [w149] -> w57
    tunnel: [w154] -> w62
    tunnel: w59 -> [w156]
    tunnel: w15 -> [w152]
    shift-right: [w148] -> _
    shift-left: w19 -> [w147]
    shift-right: [w109] -> _
    shift-left: w22 -> [w145]
    shift-right: [w144] -> _
    shift-left: w22 -> [w120]
    shift-right: [w96] -> _
    shift-left: w22 -> [w127]
    shift-right: [w140] -> _
    shift-left: 0 -> [w139]
    shift-right: [w131] -> _
    shift-left: w22 -> [w134]
    shift-right: [w132] -> _
    shift-left: 0 -> [w133]
    shift-right: [w124] -> _
    shift-left: 0.0 ("THD") -> [w123]
    shift-right: [w101] -> _
    shift-left: w22 -> [w116]
    shift-right: [w108] -> _
    shift-left: w22 -> [w115]
    shift-right: [w117] -> _
    shift-left: w22 -> [w114]
    tunnel: [w106] -> w21 mode=indexing
    shift-right: [w105] -> w20
    shift-left: w60 -> [w157]
    tunnel: w9 -> [w95]
    tunnel: w8 -> [w94]
    tunnel: w7 -> [w93]
    tunnel: w6 -> [w92]
    shift-right: [w91] -> w3
    shift-left: "Start_Amplitude(V)" -> [w90]
    i -> [w100]
    stop <- w162 stop-if-true
    w99 = 2 ("y")
    # "If the Soll_Pegel is achieved with a toleranz range \nregulating loop is ended."
    # "Finetuning Abgleich Toleranz in dB"
    # "Analysis"
    n24 = Array Size(array=w120) -> (size(s)=w112:i32)
    n25 = case shown="\"uniform white noise\", Default" w165 {
      tunnel: [w197 w214 w219 w225] -> w146
      tunnel: w164 -> [w202 w213 w218 w224]
      tunnel: [w202 w213 w218 w224] -> w158
      tunnel: w90 -> [w201 w212 w216 w220]
      tunnel: w152 -> [w199 _ _ _]
      tunnel: ["frequency" _ _ _] -> w151
      frame "uniform white noise", Default {
        n26 = Divide(x="frequency", y=w199) -> (x/y=w200:dbl)
        n27 = disable-structure shown="Enabled" {
          disable-tunnel: [w205 w211] -> w197
          disable-tunnel: w202 -> [w204 w208]
          disable-tunnel: w201 -> [w203 w206]
          disable-tunnel: w200 -> [_ w209]
          frame Disabled {
            n28 = call <vilib>:"Uniform White Noise (obs 90).vi"("amplitude"=w203, "samples"=w204) -> ("uniform white noise"=w205:dbl[])  [unwired: 1 in, 1 out]
          }
          frame Enabled {
            n29 = call <vilib>:"Sine Wave.vi"("samples"=w208, "amplitude"=w206, "frequency"=w209, "phase in"=0.0, "reset phase"=TRUE) -> ("sine wave"=w211:dbl[])  [unwired: 2 out]
          }
        }
      }
      frame "Gaussian white noise" {
        n30 = call <vilib>:"Gaussian White Noise (obs 90).vi"("standard deviation"=w212, "samples"=w213) -> ("Gaussian noise pattern"=w214:dbl[])  [unwired: 1 in, 1 out]
      }
      frame "periodic random noise" {
        n31 = Divide(x=w216, y=100.0) -> (x/y=w215:dbl)
        n32 = call <vilib>:"Periodic Random Noise.vi"("spectral amplitude"=w215, "samples"=w218) -> ("periodic random noise"=w219:dbl[])  [unwired: 1 in, 1 out]
      }
      frame "Chirp" {
        w223 = T2 0 items=["None"=0, "Hanning"=1, "Hamming"=2, "Blackman-Harris"=3, "Exact Blackman"=4, "Blackman"=5, "Flat Top"=6, "4 Term B-Harris "=7, "7 Term B-Harris"=8, "Low Sidelobe"=9, "Force - Exponential"=10, "Blackman Nuttall"=11, "Triangle"=30, "Bartlett-Hanning"=31, "Bohman"=32, "Parzen"=33, "Welch"=34, "Kaiser"=60, "Dolph-Chebyshev"=61, "Gaussian"=62] ("window")
        n33 = local write "window"(w223) -> ()
        n34 = call <vilib>:"Chirp Pattern.vi"("f2"=0.5, "f1"=0.0, "amplitude"=w220, "samples"=w224) -> ("Chirp Pattern"=w225:dbl[])  [unwired: 1 out]
      }
    }
    "Waveform Graph" <- w146
    n35 = Subtract(x=w112, y=25) -> (x-y=w113:i32)
    n36 = Greater?(x=w112, y=26) -> (0:w121:bool)
    n37 = case shown="True" w121 {
      tunnel: w120 -> [_ w181]
      tunnel: [w177 w185] -> w119
      tunnel: [w177 w184] -> w103
      tunnel: [w177 w183] -> w118
      tunnel: w113 -> [_ w180]
      frame False {
        w177 = 0.0 ("x")
      }
      frame True {
        n38 = Array Subset(array=w181, index=w180, length=25) -> (w178:dbl[])
        n39 = call <vilib>:"Std Deviation and Variance.vi"("X"=w178, "Weighting (Sample)"=enum16{"Sample", "Population"}."Population") -> ("mean"=w185:dbl, "standard deviation"=w184:dbl, "variance"=w183:dbl)
      }
    }
    "standard deviation" <- w103
    "mean" <- w119
    n40 = call "check_Coh_Faktor_past_Values.vi"("Coh Faktor Thresold in"="Coh Faktor Thresold", "Array"=w127) -> ("Boolean"=w125:bool)  [unwired: 9 in]
    n41 = Less?(x=w103, y=0.06) -> ()  [unwired: 1 out]
    n42 = call-poly <vilib>:"DAQmx Write.vi"("task/channels in"=w157, "data"=w146, "error in"=w155) -> ("task out"=w105:refnum<k21>, "error out"=w161:errorcluster)  [unwired: 10 in, 1 out]
    n43 = Equal?(x=w100, y=w99) -> (x = y?=w98:bool)
    n44 = Less?(x=w100, y=w99) -> (x < y?=w166:bool)
    n45 = Insert Into Array(array=w114, new element=w118) -> (w117:dbl[])  [unwired: 1 in]
    n46 = call-poly <vilib>:"DAQmx Read.vi"("task/channels in"=w156, "number of samples per channel"=w158, "error in"=w161) -> ("task out"=w154:refnum<k21>, "data"=w159:waveform(dbl)[], "error out"=w160:errorcluster)  [unwired: 10 in]
    n47 = case shown="False" w166 {
      tunnel: w160 -> [w269 w271]
      tunnel: w159 -> [w266 _]
      tunnel: [w253 w271] -> w150
      tunnel: w151 -> [w258 _]
      tunnel: [w247 _] -> w136
      tunnel: [w231 _] -> w124
      tunnel: [w226 0.0] -> w88
      tunnel: w95 -> [w230 _]
      tunnel: w94 -> [w229 _]
      tunnel: w93 -> [w228 _]
      tunnel: w92 -> [w227 _]
      frame False {
        # "Ist_Pegel(dBSPL) is calculated with the Fundamental detected fund. amp."
        n48 = Index Array(array=w266) -> (element #1=w265:waveform(dbl), element #2=w257:waveform(dbl))  [unwired: 2 in]
        n49 = call-poly <vilib>:"SVFA Frequency Response (Mag-Phase).vi"("stimulus signal X [EUx]"=w265, "response signal Y [EUy]"=w257, "window"=w230, "view"=w229, "error in (no error)"=w269, "averaging parameters"=w228, "restart averaging (F)"=w227) -> ("coherence"=w252:cluster{"f0":dbl, "df":dbl, "coherence":dbl[]}, "averages completed"=→"averages completed":dbl, "magnitude [dB EUy/EUx]"=w234:cluster{"f0":dbl, "df":dbl, "magnitude":dbl[]}, "phase [degrees]"=→"phase":cluster{"f0":dbl, "df":dbl, "phase":dbl[]}, "error out"=w259:errorcluster)  [unwired: 4 in, 4 out]
        "mag" <- w234
        "coherence" <- w252
        n50 = Unbundle By Name(w234) -> ("magnitude"=w233:dbl[])
        n51 = Unbundle By Name(w252) -> ("coherence"=w251:dbl[])
        n52 = call-poly <vilib>:"SVT THD and Harmonic Components.vi"("scaled signal [EU]"=w257, "maximum harmonic"="maximum harmonic", "harmonics to visualize"="harmonics to visualize", "error in (no error)"=w259, "desired units"=T7 {"THD units"=enum."%", "harmonic component amplitude units"=enum."EU peak", "detected fundamental amplitude units"=enum."EU peak"}, "expected fundamental frequency [Hz]"=w258) -> ("actual maximum harmonic"=→"actual maximum harmonic":i32, "detected fundamental\nfrequency [Hz]"=→"detected fund. freq. [Hz]":dbl, "detected fundamental\namplitude"=w231:dbl, "THD"=→"THD":dbl, "error out"=w254:errorcluster)  [unwired: 6 in, 3 out]
        "detected fund. amp." <- w231
        "fr1000Hz" <- w231
        n53 = Index Array(array=w251, index=20) -> (element=w249:dbl)
        n54 = Index Array(array=w233, index=20) -> ()  [unwired: 1 out]
        n55 = call-poly <vilib>:"SVFA Power Spectrum.vi"("scaled signal [EU]"=w257, "dB On (T)"="dB On (T)", "error in (no error)"=w254) -> ("power spectrum [dB EU]"=→"fft":cluster{"f0":dbl, "df":dbl, "magnitude":dbl[]}, "error out"=w253:errorcluster)  [unwired: 11 in, 4 out]
        n56 = Multiply(x=w231, y=1000.0 ("x")) -> (x*y=w242:dbl)
        n57 = Multiply(x=1000.0, y=w249) -> (x*y=w247:dbl)
        "coherence 2" <- w247
        "COH" <- w247
        n58 = Square Root(x=2.0) -> (sqrt(x)=w241:dbl)
        n59 = Divide(x=w242, y=w241) -> (x/y=w243:dbl)
        n60 = Divide(x=w243, y="sensitivity(mV/Pa)") -> (x/y=w238:dbl)
        "Sound Pressure (Pa)" <- w238
        n61 = Divide(x=w238, y=2e-05) -> (x/y=w239:dbl)
        n62 = Logarithm Base 10(1:w239) -> (0:w235:dbl)
        n63 = Multiply(x=w235, y=20.0 ("x")) -> (x*y=w226:dbl)
        "Ist_Pegel(dBSPL)" <- w226
        "time record 2" <- w266
        "expected fundamental frequency [Hz]" <- w258
      }
      frame True {
        # "discard first buffer (\"0\")"
      }
    }
    n64 = flat-sequence {
      tunnel: w150 -> [w195]
      tunnel: [w196] -> w148
      tunnel: [w195] -> w149
      frame #0 {
        n65 = Tick Count (ms)() -> (millisecond timer value=w196:u32)
      }
    }
    n66 = Unbundle By Name(w150) -> ("status"=w163:bool)
    n67 = Less?(x=w136, y="Coh Faktor Thresold") -> (x < y?=w129:bool)
    n68 = Subtract(x="Soll_Pegel(dBSPL)", y=w88) -> (x-y=w86:dbl)
    n69 = Or(x=w129, y=w125) -> (x .or. y?=w128:bool)
    n70 = Absolute Value(x=w86) -> (abs(x)=w85:dbl)
    n71 = case shown="True" w128 {
      tunnel: w123 -> [w187 w188]
      tunnel: [w187 w188] -> w135
      tunnel: w133 -> [w186 w191]
      tunnel: [w186 w190] -> w132
      tunnel: w125 -> [_ w189]
      frame False {
      }
      frame True {
        n72 = case shown="False" w189 {
          tunnel: w191 -> [w193 w194]
          tunnel: [w192 w194] -> w190
          frame False {
            n73 = Increment(x=w193) -> (x+1=w192:i32)
          }
          frame True {
          }
        }
      }
    }
    "Big Sound Disturbances detected" <- w132
    n74 = Less?(x=w85, y=0.1) -> (x < y?=w84:bool)
    n75 = Subtract(x=w148, y=w147) -> (x-y=w106:u32)
    "loop time(ms)" <- w106
    n76 = Compound Arithmetic op=OR(w163, "stop", w84) -> (w162:bool)
    n77 = Divide(x=w106, y=u32 1000) -> (x/y=w138:dbl)
    n78 = Add(x=w139, y=w138) -> (x+y=w140:dbl)
    n79 = Insert Into Array(array=w115, new element=w103) -> (w108:dbl[])  [unwired: 1 in]
    n80 = Insert Into Array(array=w134, new element=w135) -> (w131:dbl[])  [unwired: 1 in]
    n81 = Insert Into Array(array=w127, new element=w136) -> (w97:dbl[])  [unwired: 1 in]
    n82 = Insert Into Array(array=w145, new element=w140) -> (w109:dbl[])  [unwired: 1 in]
    n83 = Insert Into Array(array=w120, new element=w124) -> (w144:dbl[])  [unwired: 1 in]
    n84 = Insert Into Array(array=w116, new element=w88) -> (w102:dbl[])  [unwired: 1 in]
    n85 = Bundle(w109, w131) -> (→"Filtered FR_Time Chart":cluster{dbl[], dbl[]})  [unwired: 1 in]
    n86 = Bundle(w109, w97) -> (w142:cluster{dbl[], dbl[]})  [unwired: 1 in]
    n87 = Bundle(w109, w108) -> ()  [unwired: 1 in, 1 out]
    n88 = Bundle(w109, w144) -> (w143:cluster{dbl[], dbl[]})  [unwired: 1 in]
    n89 = Bundle(w109, w102) -> (w110:cluster{dbl[], dbl[]})  [unwired: 1 in]
    n90 = Build Array(w143, w142) -> (→"Coh_FR_Time Chart":cluster{dbl[], dbl[]}[])
    n91 = case shown="True" w98 {
      tunnel: w102 -> [w168 w176]
      tunnel: [w168 w173] -> w101
      tunnel: w97 -> [w167 w170]
      tunnel: [w167 w169] -> w96
      frame False {
      }
      frame True {
        n92 = Delete From Array(array=w170, length=2, index=0) -> (array with subset deleted=w169:dbl[])  [unwired: 1 out]
        n93 = Delete From Array(array=w176, length=2, index=0) -> (array with subset deleted=w173:dbl[])  [unwired: 1 out]
      }
    }
    n94 = Build Array(w110) -> (→"Ist_Pegel(dBSPL) Time Chart":cluster{dbl[], dbl[]}[])
    n95 = call "Amplitude_Calculation_for_finetuning.vi"("Amplitude_In(V)"=w90, "Ist_Pegel(dBSPL)"=w88, "Soll_Pegel(dBSPL)"="Soll_Pegel(dBSPL)") -> ("Amplitude_Out(V)"=w91:dbl)  [unwired: 8 in]
  }
  "Array" <- w21
  "End_Amplitude(V)" <- w3
  n96 = call <vilib>:"DAQmx Clear Task.vi"("task in"=w62, "error in"=w57) -> ("error out"=w56:errorcluster)  [unwired: 13 in]
  n97 = call-poly <vilib>:"DAQmx Write.vi"("task/channels in"=w20, "data"=w55, "error in"=w56) -> ("task out"=w54:refnum<k21>, "error out"=w53:errorcluster)  [unwired: 10 in, 1 out]
  n98 = stacked-sequence {
    tunnel: w53 -> [w273]
    tunnel: [w273] -> w52
    tunnel: w48 -> [w272]
    frame #0 {
      n99 = Wait (ms)(milliseconds to wait=w272) -> ()  [unwired: 1 out]
    }
  }
  n100 = call <vilib>:"DAQmx Clear Task.vi"("task in"=w54, "error in"=w52) -> ("error out"=→"error out":errorcluster)  [unwired: 13 in]
